vi "SLSC Create Tree Control from EDS datatype.vi"(7 "Property Tree":refnum<vi>, 8 "error in (no error)":errorcluster, 9 "Channel Values":dbl[](array[numeric]), 10 "Properties to enable":string[](array[string]), 11 "SLSC EDS module":T3) -> (0 "error out":errorcluster, 1 "Enum Strings":cluster{"name":string, string}[](array[cluster]), 2 "Enums":T1[](array[typedef]), 3 "SLSC Output Tree":T2(array[cluster])=[{"Left Cell String"="SLSC-12001-030EE1BC-Mod8", "Child Text"=[], "Child Tag"="Device", "Item Indent"=0, "Child Only?"=FALSE, "Glyph Index"=28}, {"Left Cell String"="Commands", "Child Text"=[], "Child Tag"="Device/Commands", "Item Indent"=1, "Child Only?"=FALSE, "Glyph Index"=35}, {"Left Cell String"="NI.UpdateChannelConfiguration", "Child Text"=["", "", "", "", "", "", "Command..NI.UpdateChannelConfiguration", "Command to complete updating physical channel properties", "This command enables simultaneous updating of the functional state of the module's physical channel configuration. Simultaneous updating of the physical channels' properties prevents the register write commit order from creating unexpected channel configuration states. Run this command to make changes to physical channels' properties take effect."], "Child Tag"="Device/Commands/NI.UpdateChannelConfiguration", "Item Indent"=2, "Child Only?"=FALSE, "Glyph Index"=4}, {"Left Cell String"="NI.UpdateTestMode", "Child Text"=["", "", "", "", "", "", "Command..NI.UpdateTestMode", "Command to complete updating Test Mode properties", "This command enable simultaneous updating of the functional state of the module's Test Mode configuration. Run this command to make changes to Test Mode properties take effect."], "Child Tag"="Device/Commands/NI.UpdateTestMode", "Item Indent"=2, "Child Only?"=FALSE, "Glyph Index"=4}, {"Left Cell String"="NI.Acknowledge24VPowerFailed", "Child Text"=["", "", "", "", "", "", "Command..NI.Acknowledge24VPowerFailed", "Command to acknowledge a latched 24V power failure status", "This command tries to clear the module's latched true state for the NI.Status24V_PowerFailed property. This command will have no effect on the latched state if the NI.Status24V_PowerGood property is still false."], "Child Tag"="Device/Commands/NI.Acknowledge24VPowerFailed", "Item Indent"=2, "Child Only?"=FALSE, "Glyph Index"=4}, {"Left Cell String"="Properties", "Child Text"=[], "Child Tag"="Device/Properties", "Item Indent"=1, "Child Only?"=FALSE, "Glyph Index"=36}, {"Left Cell String"="NI.ModuleControllerVersion", "Child Text"=["17022812", "Read Only", "U32", "", "", "", "[3.860173E+8].R.U32..NI.ModuleControllerVersion", "Module Controller Version", "The version is the timestamp, in hexadecimal format, of the time the Module Controller was compiled."], "Child Tag"="Device/Properties/NI.ModuleControllerVersion", "Item Indent"=2, "Child Only?"=FALSE, "Glyph Index"=8}, {"Left Cell String"="NI.RearBufferState", "Child Text"=["0", "Read Only", "U32", "", "", "", "[0].R.U32..NI.RearBufferState", "Logic state of all rear I/O connector input buffers", "Reading this property retrieves the current logic state of the rear I/O connector input buffers. This retrieval is controlled through the software system so the actual sampling time of the inputs is not deterministic. The value at each bit position is a function of the logic state at the XJ2 pin and the corresponding line's direction and enable configuration. An enabled line configured as an input will drive the rear I/O connector input buffer to the same state as detected at the front I/O connector input buffer."], "Child Tag"="Device/Properties/NI.RearBufferState", "Item Indent"=2, "Child Only?"=FALSE, "Glyph Index"=8}, {"Left Cell String"="NI.FrontBufferState", "Child Text"=["0", "Read Only", "U32", "", "", "", "[0].R.U32..NI.FrontBufferState", "Logic state of all front I/O connector input buffers", "Reading this property retrieves the current logic state of the front I/O connector input buffers. This retrieval is controlled through the software system so the actual sampling time of the inputs is not deterministic. The value at each bit position is a function of the voltage at the module DSUB pin and the bank range and threshold configuration. An enabled line configured as an output may drive the front I/O connector input buffer to a specific voltage, depending on the bank supply voltage configuration, the line's output topology, and the line's logic state from the rear I/O connector input buffer."], "Child Tag"="Device/Properties/NI.FrontBufferState", "Item Indent"=2, "Child Only?"=FALSE, "Glyph Index"=8}, {"Left Cell String"="NI.Status24VPowerFailed", "Child Text"=["False", "Read Only", "Bool", "", "", "", "[0].R.Bool..NI.Status24VPowerFailed", "State of the latched failure status of the module's 24V rail from the SLSC Interface", "When the NI.Status24V_PowerGood becomes false, this property latches as true until it is reset by the NI.Status24V_FaultAcknowledge command is sent after NI.Status24V_PowerGood returns to true. If this property is true, then the supply voltage selection for both banks of the module has been forced off for a nonzero duration."], "Child Tag"="Device/Properties/NI.Status24VPowerFailed", "Item Indent"=2, "Child Only?"=FALSE, "Glyph Index"=8}, {"Left Cell String"="NI.Status24VPowerGood", "Child Text"=["True", "Read Only", "Bool", "", "", "", "[1].R.Bool..NI.Status24VPowerGood", "State of the 24V rail on the module from the SLSC Interface", "When the 24V rail from the SLSC Interface drops below the safe operating range for the module, this property is set to false. Simultaneously, to protect the module's output circuitry and to prevent the module front I/O connector outputs from glitching high, the supply voltage selection for both banks is forced off until the 24V rail recovers and is stable."], "Child Tag"="Device/Properties/NI.Status24VPowerGood", "Item Indent"=2, "Child Only?"=FALSE, "Glyph Index"=8}, {"Left Cell String"="NI.Status3_3VPowerGood", "Child Text"=["True", "Read Only", "Bool", "", "", "", "[1].R.Bool..NI.Status3_3VPowerGood", "State of the 3.3V rail from the SLSC Interface on the module", "This property will always be true on a correctly functioning module because the module CPLD requires the 3.3V rail from the SLSC Interface to operate."], "Child Tag"="Device/Properties/NI.Status3_3VPowerGood", "Item Indent"=2, "Child Only?"=FALSE, "Glyph Index"=8}, {"Left Cell String"="NI.TestModeEnable", "Child Text"=["False", "Read/Write", "Bool", "", "", "", "[0].RW.Bool..NI.TestModeEnable", "Enable for Test Mode", "Enable state for the module's Test Mode. When Test Mode is enabled, the module will output the values from the NI.TestModeValue property on the corresponding lines. Each line's respective direction and enable configuration will still apply when Test Mode is active. The data source of the lines is the only change when Test Mode is active. Changes to this property take effect after running the NI.TestModeUpdate command."], "Child Tag"="Device/Properties/NI.TestModeEnable", "Item Indent"=2, "Child Only?"=FALSE, "Glyph Index"=9}, {"Left Cell String"="NI.TestModeValue", "Child Text"=["0", "Read/Write", "U32", "", "", "", "[0].RW.U32..NI.TestModeValue", "Output logic states for use during Test Mode", "Output logic states for the module for use during Test Mode. The logic state corresponding to each line may be set independently of the other states. Changes to this property take effect after running the NI.TestModeUpdate command."], "Child Tag"="Device/Properties/NI.TestModeValue", "Item Indent"=2, "Child Only?"=FALSE, "Glyph Index"=9}, {"Left Cell String"="SLSC-12001-030EE1BC-Mod8/bank0", "Child Text"=[], "Child Tag"="Physical Channel/bank0", "Item Indent"=1, "Child Only?"=FALSE, "Glyph Index"=31}, {"Left Cell String"="Commands", "Child Text"=[], "Child Tag"="Physical Channel/bank0/Commands", "Item Indent"=2, "Child Only?"=FALSE, "Glyph Index"=35}, {"Left Cell String"="Properties", "Child Text"=[], "Child Tag"="Physical Channel/bank0/Properties", "Item Indent"=2, "Child Only?"=FALSE, "Glyph Index"=36}, {"Left Cell String"="NI.VsupSelect", "Child Text"=["[0]Vsup_Off", "Read/Write", "I32", "Enum", "NI.VsupSource", "[0]Vsup_Off;[1]Vsup_0;[2]Vsup_1;", "[0].RW.I32.bank0.NI.VsupSelect", "Voltage source selection", "Voltage source selection for this bank. Changes to this property take effect after running the NI.ChannelConfigurationUpdate command."], "Child Tag"="Physical Channel/bank0/Properties/NI.VsupSelect", "Item Indent"=3, "Child Only?"=FALSE, "Glyph Index"=9}, {"Left Cell String"="NI.RangeEnable5V", "Child Text"=["False", "Read/Write", "Bool", "", "", "", "[0].RW.Bool.bank0.NI.RangeEnable5V", "Voltage range selection", "Enable state for this bank's voltage range. When enabled, this bank uses the NI.InputThreshold5V for the input threshold. When disabled, this bank uses the NI.InputThreshold33V for the input threshold. Changes to this property take effect after running the NI.ChannelConfigurationUpdate command."], "Child Tag"="Physical Channel/bank0/Properties/NI.RangeEnable5V", "Item Indent"=3, "Child Only?"=FALSE, "Glyph Index"=9}, {"Left Cell String"="NI.InputThreshold5V", "Child Text"=["0.7", "Read/Write", "DBL", "", "", "", "[0.7].RW.DBL.bank0.NI.InputThreshold5V", "Input threshold voltage for the 5 V range", "Input threshold voltage for this bank when its NI.RangeEnable5V is true. Changes to this property take effect after running the NI.ChannelConfigurationUpdate command."], "Child Tag"="Physical Channel/bank0/Properties/NI.InputThreshold5V", "Item Indent"=3, "Child Only?"=FALSE, "Glyph Index"=9}, {"Left Cell String"="NI.InputThreshold33V", "Child Text"=["3.706", "Read/Write", "DBL", "", "", "", "[3.706].RW.DBL.bank0.NI.InputThreshold33V", "Input threshold voltage for the 33 V range", "Input threshold voltage for this bank when its NI.RangeEnable5V is false. Changes to this property take effect after running the NI.ChannelConfigurationUpdate command."], "Child Tag"="Physical Channel/bank0/Properties/NI.InputThreshold33V", "Item Indent"=3, "Child Only?"=FALSE, "Glyph Index"=9}, {"Left Cell String"="SLSC-12001-030EE1BC-Mod8/bank1", "Child Text"=[], "Child Tag"="Physical Channel/bank1", "Item Indent"=1, "Child Only?"=FALSE, "Glyph Index"=31}, {"Left Cell String"="Commands", "Child Text"=[], "Child Tag"="Physical Channel/bank1/Commands", "Item Indent"=2, "Child Only?"=FALSE, "Glyph Index"=35}, {"Left Cell String"="Properties", "Child Text"=[], "Child Tag"="Physical Channel/bank1/Properties", "Item Indent"=2, "Child Only?"=FALSE, "Glyph Index"=36}, {"Left Cell String"="NI.VsupSelect", "Child Text"=["[0]Vsup_Off", "Read/Write", "I32", "Enum", "NI.VsupSource", "[0]Vsup_Off;[1]Vsup_0;[2]Vsup_1;", "[0].RW.I32.bank1.NI.VsupSelect", "Voltage source selection", "Voltage source selection for this bank. Changes to this property take effect after running the NI.ChannelConfigurationUpdate command."], "Child Tag"="Physical Channel/bank1/Properties/NI.VsupSelect", "Item Indent"=3, "Child Only?"=FALSE, "Glyph Index"=9}, {"Left Cell String"="NI.RangeEnable5V", "Child Text"=["False", "Read/Write", "Bool", "", "", "", "[0].RW.Bool.bank1.NI.RangeEnable5V", "Voltage range selection", "Enable state for this bank's voltage range. When enabled, this bank uses the NI.InputThreshold5V for the input threshold. When disabled, this bank uses the NI.InputThreshold33V for the input threshold. Changes to this property take effect after running the NI.ChannelConfigurationUpdate command."], "Child Tag"="Physical Channel/bank1/Properties/NI.RangeEnable5V", "Item Indent"=3, "Child Only?"=FALSE, "Glyph Index"=9}, {"Left Cell String"="NI.InputThreshold5V", "Child Text"=["0.7", "Read/Write", "DBL", "", "", "", "[0.7].RW.DBL.bank1.NI.InputThreshold5V", "Input threshold voltage for the 5 V range", "Input threshold voltage for this bank when its NI.RangeEnable5V is true. Changes to this property take effect after running the NI.ChannelConfigurationUpdate command."], "Child Tag"="Physical Channel/bank1/Properties/NI.InputThreshold5V", "Item Indent"=3, "Child Only?"=FALSE, "Glyph Index"=9}, {"Left Cell String"="NI.InputThreshold33V", "Child Text"=["3.706", "Read/Write", "DBL", "", "", "", "[3.706].RW.DBL.bank1.NI.InputThreshold33V", "Input threshold voltage for the 33 V range", "Input threshold voltage for this bank when its NI.RangeEnable5V is false. Changes to this property take effect after running the NI.ChannelConfigurationUpdate command."], "Child Tag"="Physical Channel/bank1/Properties/NI.InputThreshold33V", "Item Indent"=3, "Child Only?"=FALSE, "Glyph Index"=9}, {"Left Cell String"="SLSC-12001-030EE1BC-Mod8/port0/line0", "Child Text"=[], "Child Tag"="Physical Channel/port0/line0", "Item Indent"=1, "Child Only?"=FALSE, "Glyph Index"=31}, {"Left Cell String"="Commands", "Child Text"=[], "Child Tag"="Physical Channel/port0/line0/Commands", "Item Indent"=2, "Child Only?"=FALSE, "Glyph Index"=35}, {"Left Cell String"="Properties", "Child Text"=[], "Child Tag"="Physical Channel/port0/line0/Properties", "Item Indent"=2, "Child Only?"=FALSE, "Glyph Index"=36}, {"Left Cell String"="NI.Line.Index", "Child Text"=["0", "Read Only", "U32", "", "", "", "[0].R.U32.port0/line0.NI.Line.Index", "Overall index of this DIO line in the module", "This is the index of this DIO line for the aggregate module properties: NI.FrontInputBufferState, NI.RearInputBufferState, and NI.TestModeValue."], "Child Tag"="Physical Channel/port0/line0/Properties/NI.Line.Index", "Item Indent"=3, "Child Only?"=FALSE, "Glyph Index"=8}, {"Left Cell String"="NI.Line.Direction", "Child Text"=["[0]Input", "Read/Write", "I32", "Enum", "NI.Line.Direction", "[0]Input;[1]Output_Source;[2]Output_Sink;[3]Output_PushPull;", "[0].RW.I32.port0/line0.NI.Line.Direction", "DIO line direction", "Line signal flow direction through the module, relative to the front I/O connector. This property is only used when the NI.ChannelEnable for this line is set to true. Changes to this property take effect after running the NI.ChannelConfigurationUpdate command."], "Child Tag"="Physical Channel/port0/line0/Properties/NI.Line.Direction", "Item Indent"=3, "Child Only?"=FALSE, "Glyph Index"=9}, {"Left Cell String"="NI.Line.Enable", "Child Text"=["False", "Read/Write", "Bool", "", "", "", "[0].RW.Bool.port0/line0.NI.Line.Enable", "DIO line output enable", "DIO output enable for one line. When a line is enabled, the input and output buffers for the front I/O connector and the rear I/O connector of the line are configured based on the NI.Line.Direction property. When a line is not enabled, the buffers for both the front I/O connector and the rear I/O connector are configured as inputs. Changes to this property take effect after running the NI.ChannelConfigurationUpdate command."], "Child Tag"="Physical Channel/port0/line0/Properties/NI.Line.Enable", "Item Indent"=3, "Child Only?"=FALSE, "Glyph Index"=9}, {"Left Cell String"="SLSC-12001-030EE1BC-Mod8/port0/line1", "Child Text"=[], "Child Tag"="Physical Channel/port0/line1", "Item Indent"=1, "Child Only?"=FALSE, "Glyph Index"=31}, {"Left Cell String"="Commands", "Child Text"=[], "Child Tag"="Physical Channel/port0/line1/Commands", "Item Indent"=2, "Child Only?"=FALSE, "Glyph Index"=35}, {"Left Cell String"="Properties", "Child Text"=[], "Child Tag"="Physical Channel/port0/line1/Properties", "Item Indent"=2, "Child Only?"=FALSE, "Glyph Index"=36}, {"Left Cell String"="NI.Line.Index", "Child Text"=["1", "Read Only", "U32", "", "", "", "[1].R.U32.port0/line1.NI.Line.Index", "Overall index of this DIO line in the module", "This is the index of this DIO line for the aggregate module properties: NI.FrontInputBufferState, NI.RearInputBufferState, and NI.TestModeValue."], "Child Tag"="Physical Channel/port0/line1/Properties/NI.Line.Index", "Item Indent"=3, "Child Only?"=FALSE, "Glyph Index"=8}, {"Left Cell String"="NI.Line.Direction", "Child Text"=["[0]Input", "Read/Write", "I32", "Enum", "NI.Line.Direction", "[0]Input;[1]Output_Source;[2]Output_Sink;[3]Output_PushPull;", "[0].RW.I32.port0/line1.NI.Line.Direction", "DIO line direction", "Line signal flow direction through the module, relative to the front I/O connector. This property is only used when the NI.ChannelEnable for this line is set to true. Changes to this property take effect after running the NI.ChannelConfigurationUpdate command."], "Child Tag"="Physical Channel/port0/line1/Properties/NI.Line.Direction", "Item Indent"=3, "Child Only?"=FALSE, "Glyph Index"=9}, {"Left Cell String"="NI.Line.Enable", "Child Text"=["False", "Read/Write", "Bool", "", "", "", "[0].RW.Bool.port0/line1.NI.Line.Enable", "DIO line output enable", "DIO output enable for one line. When a line is enabled, the input and output buffers for the front I/O connector and the rear I/O connector of the line are configured based on the NI.Line.Direction property. When a line is not enabled, the buffers for both the front I/O connector and the rear I/O connector are configured as inputs. Changes to this property take effect after running the NI.ChannelConfigurationUpdate command."], "Child Tag"="Physical Channel/port0/line1/Properties/NI.Line.Enable", "Item Indent"=3, "Child Only?"=FALSE, "Glyph Index"=9}, {"Left Cell String"="SLSC-12001-030EE1BC-Mod8/port0/line2", "Child Text"=[], "Child Tag"="Physical Channel/port0/line2", "Item Indent"=1, "Child Only?"=FALSE, "Glyph Index"=31}, {"Left Cell String"="Commands", "Child Text"=[], "Child Tag"="Physical Channel/port0/line2/Commands", "Item Indent"=2, "Child Only?"=FALSE, "Glyph Index"=35}, {"Left Cell String"="Properties", "Child Text"=[], "Child Tag"="Physical Channel/port0/line2/Properties", "Item Indent"=2, "Child Only?"=FALSE, "Glyph Index"=36}, {"Left Cell String"="NI.Line.Index", "Child Text"=["2", "Read Only", "U32", "", "", "", "[2].R.U32.port0/line2.NI.Line.Index", "Overall index of this DIO line in the module", "This is the index of this DIO line for the aggregate module properties: NI.FrontInputBufferState, NI.RearInputBufferState, and NI.TestModeValue."], "Child Tag"="Physical Channel/port0/line2/Properties/NI.Line.Index", "Item Indent"=3, "Child Only?"=FALSE, "Glyph Index"=8}, {"Left Cell String"="NI.Line.Direction", "Child Text"=["[0]Input", "Read/Write", "I32", "Enum", "NI.Line.Direction", "[0]Input;[1]Output_Source;[2]Output_Sink;[3]Output_PushPull;", "[0].RW.I32.port0/line2.NI.Line.Direction", "DIO line direction", "Line signal flow direction through the module, relative to the front I/O connector. This property is only used when the NI.ChannelEnable for this line is set to true. Changes to this property take effect after running the NI.ChannelConfigurationUpdate command."], "Child Tag"="Physical Channel/port0/line2/Properties/NI.Line.Direction", "Item Indent"=3, "Child Only?"=FALSE, "Glyph Index"=9}, {"Left Cell String"="NI.Line.Enable", "Child Text"=["False", "Read/Write", "Bool", "", "", "", "[0].RW.Bool.port0/line2.NI.Line.Enable", "DIO line output enable", "DIO output enable for one line. When a line is enabled, the input and output buffers for the front I/O connector and the rear I/O connector of the line are configured based on the NI.Line.Direction property. When a line is not enabled, the buffers for both the front I/O connector and the rear I/O connector are configured as inputs. Changes to this property take effect after running the NI.ChannelConfigurationUpdate command."], "Child Tag"="Physical Channel/port0/line2/Properties/NI.Line.Enable", "Item Indent"=3, "Child Only?"=FALSE, "Glyph Index"=9}, {"Left Cell String"="SLSC-12001-030EE1BC-Mod8/port0/line3", "Child Text"=[], "Child Tag"="Physical Channel/port0/line3", "Item Indent"=1, "Child Only?"=FALSE, "Glyph Index"=31}, {"Left Cell String"="Commands", "Child Text"=[], "Child Tag"="Physical Channel/port0/line3/Commands", "Item Indent"=2, "Child Only?"=FALSE, "Glyph Index"=35}, {"Left Cell String"="Properties", "Child Text"=[], "Child Tag"="Physical Channel/port0/line3/Properties", "Item Indent"=2, "Child Only?"=FALSE, "Glyph Index"=36}, {"Left Cell String"="NI.Line.Index", "Child Text"=["3", "Read Only", "U32", "", "", "", "[3].R.U32.port0/line3.NI.Line.Index", "Overall index of this DIO line in the module", "This is the index of this DIO line for the aggregate module properties: NI.FrontInputBufferState, NI.RearInputBufferState, and NI.TestModeValue."], "Child Tag"="Physical Channel/port0/line3/Properties/NI.Line.Index", "Item Indent"=3, "Child Only?"=FALSE, "Glyph Index"=8}, {"Left Cell String"="NI.Line.Direction", "Child Text"=["[0]Input", "Read/Write", "I32", "Enum", "NI.Line.Direction", "[0]Input;[1]Output_Source;[2]Output_Sink;[3]Output_PushPull;", "[0].RW.I32.port0/line3.NI.Line.Direction", "DIO line direction", "Line signal flow direction through the module, relative to the front I/O connector. This property is only used when the NI.ChannelEnable for this line is set to true. Changes to this property take effect after running the NI.ChannelConfigurationUpdate command."], "Child Tag"="Physical Channel/port0/line3/Properties/NI.Line.Direction", "Item Indent"=3, "Child Only?"=FALSE, "Glyph Index"=9}, {"Left Cell String"="NI.Line.Enable", "Child Text"=["False", "Read/Write", "Bool", "", "", "", "[0].RW.Bool.port0/line3.NI.Line.Enable", "DIO line output enable", "DIO output enable for one line. When a line is enabled, the input and output buffers for the front I/O connector and the rear I/O connector of the line are configured based on the NI.Line.Direction property. When a line is not enabled, the buffers for both the front I/O connector and the rear I/O connector are configured as inputs. Changes to this property take effect after running the NI.ChannelConfigurationUpdate command."], "Child Tag"="Physical Channel/port0/line3/Properties/NI.Line.Enable", "Item Indent"=3, "Child Only?"=FALSE, "Glyph Index"=9}, {"Left Cell String"="SLSC-12001-030EE1BC-Mod8/port0/line4", "Child Text"=[], "Child Tag"="Physical Channel/port0/line4", "Item Indent"=1, "Child Only?"=FALSE, "Glyph Index"=31}, {"Left Cell String"="Commands", "Child Text"=[], "Child Tag"="Physical Channel/port0/line4/Commands", "Item Indent"=2, "Child Only?"=FALSE, "Glyph Index"=35}, {"Left Cell String"="Properties", "Child Text"=[], "Child Tag"="Physical Channel/port0/line4/Properties", "Item Indent"=2, "Child Only?"=FALSE, "Glyph Index"=36}, {"Left Cell String"="NI.Line.Index", "Child Text"=["4", "Read Only", "U32", "", "", "", "[4].R.U32.port0/line4.NI.Line.Index", "Overall index of this DIO line in the module", "This is the index of this DIO line for the aggregate module properties: NI.FrontInputBufferState, NI.RearInputBufferState, and NI.TestModeValue."], "Child Tag"="Physical Channel/port0/line4/Properties/NI.Line.Index", "Item Indent"=3, "Child Only?"=FALSE, "Glyph Index"=8}, {"Left Cell String"="NI.Line.Direction", "Child Text"=["[0]Input", "Read/Write", "I32", "Enum", "NI.Line.Direction", "[0]Input;[1]Output_Source;[2]Output_Sink;[3]Output_PushPull;", "[0].RW.I32.port0/line4.NI.Line.Direction", "DIO line direction", "Line signal flow direction through the module, relative to the front I/O connector. This property is only used when the NI.ChannelEnable for this line is set to true. Changes to this property take effect after running the NI.ChannelConfigurationUpdate command."], "Child Tag"="Physical Channel/port0/line4/Properties/NI.Line.Direction", "Item Indent"=3, "Child Only?"=FALSE, "Glyph Index"=9}, {"Left Cell String"="NI.Line.Enable", "Child Text"=["False", "Read/Write", "Bool", "", "", "", "[0].RW.Bool.port0/line4.NI.Line.Enable", "DIO line output enable", "DIO output enable for one line. When a line is enabled, the input and output buffers for the front I/O connector and the rear I/O connector of the line are configured based on the NI.Line.Direction property. When a line is not enabled, the buffers for both the front I/O connector and the rear I/O connector are configured as inputs. Changes to this property take effect after running the NI.ChannelConfigurationUpdate command."], "Child Tag"="Physical Channel/port0/line4/Properties/NI.Line.Enable", "Item Indent"=3, "Child Only?"=FALSE, "Glyph Index"=9}, {"Left Cell String"="SLSC-12001-030EE1BC-Mod8/port0/line5", "Child Text"=[], "Child Tag"="Physical Channel/port0/line5", "Item Indent"=1, "Child Only?"=FALSE, "Glyph Index"=31}, {"Left Cell String"="Commands", "Child Text"=[], "Child Tag"="Physical Channel/port0/line5/Commands", "Item Indent"=2, "Child Only?"=FALSE, "Glyph Index"=35}, {"Left Cell String"="Properties", "Child Text"=[], "Child Tag"="Physical Channel/port0/line5/Properties", "Item Indent"=2, "Child Only?"=FALSE, "Glyph Index"=36}, {"Left Cell String"="NI.Line.Index", "Child Text"=["5", "Read Only", "U32", "", "", "", "[5].R.U32.port0/line5.NI.Line.Index", "Overall index of this DIO line in the module", "This is the index of this DIO line for the aggregate module properties: NI.FrontInputBufferState, NI.RearInputBufferState, and NI.TestModeValue."], "Child Tag"="Physical Channel/port0/line5/Properties/NI.Line.Index", "Item Indent"=3, "Child Only?"=FALSE, "Glyph Index"=8}, {"Left Cell String"="NI.Line.Direction", "Child Text"=["[0]Input", "Read/Write", "I32", "Enum", "NI.Line.Direction", "[0]Input;[1]Output_Source;[2]Output_Sink;[3]Output_PushPull;", "[0].RW.I32.port0/line5.NI.Line.Direction", "DIO line direction", "Line signal flow direction through the module, relative to the front I/O connector. This property is only used when the NI.ChannelEnable for this line is set to true. Changes to this property take effect after running the NI.ChannelConfigurationUpdate command."], "Child Tag"="Physical Channel/port0/line5/Properties/NI.Line.Direction", "Item Indent"=3, "Child Only?"=FALSE, "Glyph Index"=9}, {"Left Cell String"="NI.Line.Enable", "Child Text"=["False", "Read/Write", "Bool", "", "", "", "[0].RW.Bool.port0/line5.NI.Line.Enable", "DIO line output enable", "DIO output enable for one line. When a line is enabled, the input and output buffers for the front I/O connector and the rear I/O connector of the line are configured based on the NI.Line.Direction property. When a line is not enabled, the buffers for both the front I/O connector and the rear I/O connector are configured as inputs. Changes to this property take effect after running the NI.ChannelConfigurationUpdate command."], "Child Tag"="Physical Channel/port0/line5/Properties/NI.Line.Enable", "Item Indent"=3, "Child Only?"=FALSE, "Glyph Index"=9}, {"Left Cell String"="SLSC-12001-030EE1BC-Mod8/port0/line6", "Child Text"=[], "Child Tag"="Physical Channel/port0/line6", "Item Indent"=1, "Child Only?"=FALSE, "Glyph Index"=31}, {"Left Cell String"="Commands", "Child Text"=[], "Child Tag"="Physical Channel/port0/line6/Commands", "Item Indent"=2, "Child Only?"=FALSE, "Glyph Index"=35}, {"Left Cell String"="Properties", "Child Text"=[], "Child Tag"="Physical Channel/port0/line6/Properties", "Item Indent"=2, "Child Only?"=FALSE, "Glyph Index"=36}, {"Left Cell String"="NI.Line.Index", "Child Text"=["6", "Read Only", "U32", "", "", "", "[6].R.U32.port0/line6.NI.Line.Index", "Overall index of this DIO line in the module", "This is the index of this DIO line for the aggregate module properties: NI.FrontInputBufferState, NI.RearInputBufferState, and NI.TestModeValue."], "Child Tag"="Physical Channel/port0/line6/Properties/NI.Line.Index", "Item Indent"=3, "Child Only?"=FALSE, "Glyph Index"=8}, {"Left Cell String"="NI.Line.Direction", "Child Text"=["[0]Input", "Read/Write", "I32", "Enum", "NI.Line.Direction", "[0]Input;[1]Output_Source;[2]Output_Sink;[3]Output_PushPull;", "[0].RW.I32.port0/line6.NI.Line.Direction", "DIO line direction", "Line signal flow direction through the module, relative to the front I/O connector. This property is only used when the NI.ChannelEnable for this line is set to true. Changes to this property take effect after running the NI.ChannelConfigurationUpdate command."], "Child Tag"="Physical Channel/port0/line6/Properties/NI.Line.Direction", "Item Indent"=3, "Child Only?"=FALSE, "Glyph Index"=9}, {"Left Cell String"="NI.Line.Enable", "Child Text"=["False", "Read/Write", "Bool", "", "", "", "[0].RW.Bool.port0/line6.NI.Line.Enable", "DIO line output enable", "DIO output enable for one line. When a line is enabled, the input and output buffers for the front I/O connector and the rear I/O connector of the line are configured based on the NI.Line.Direction property. When a line is not enabled, the buffers for both the front I/O connector and the rear I/O connector are configured as inputs. Changes to this property take effect after running the NI.ChannelConfigurationUpdate command."], "Child Tag"="Physical Channel/port0/line6/Properties/NI.Line.Enable", "Item Indent"=3, "Child Only?"=FALSE, "Glyph Index"=9}, {"Left Cell String"="SLSC-12001-030EE1BC-Mod8/port0/line7", "Child Text"=[], "Child Tag"="Physical Channel/port0/line7", "Item Indent"=1, "Child Only?"=FALSE, "Glyph Index"=31}, {"Left Cell String"="Commands", "Child Text"=[], "Child Tag"="Physical Channel/port0/line7/Commands", "Item Indent"=2, "Child Only?"=FALSE, "Glyph Index"=35}, {"Left Cell String"="Properties", "Child Text"=[], "Child Tag"="Physical Channel/port0/line7/Properties", "Item Indent"=2, "Child Only?"=FALSE, "Glyph Index"=36}, {"Left Cell String"="NI.Line.Index", "Child Text"=["7", "Read Only", "U32", "", "", "", "[7].R.U32.port0/line7.NI.Line.Index", "Overall index of this DIO line in the module", "This is the index of this DIO line for the aggregate module properties: NI.FrontInputBufferState, NI.RearInputBufferState, and NI.TestModeValue."], "Child Tag"="Physical Channel/port0/line7/Properties/NI.Line.Index", "Item Indent"=3, "Child Only?"=FALSE, "Glyph Index"=8}, {"Left Cell String"="NI.Line.Direction", "Child Text"=["[0]Input", "Read/Write", "I32", "Enum", "NI.Line.Direction", "[0]Input;[1]Output_Source;[2]Output_Sink;[3]Output_PushPull;", "[0].RW.I32.port0/line7.NI.Line.Direction", "DIO line direction", "Line signal flow direction through the module, relative to the front I/O connector. This property is only used when the NI.ChannelEnable for this line is set to true. Changes to this property take effect after running the NI.ChannelConfigurationUpdate command."], "Child Tag"="Physical Channel/port0/line7/Properties/NI.Line.Direction", "Item Indent"=3, "Child Only?"=FALSE, "Glyph Index"=9}, {"Left Cell String"="NI.Line.Enable", "Child Text"=["False", "Read/Write", "Bool", "", "", "", "[0].RW.Bool.port0/line7.NI.Line.Enable", "DIO line output enable", "DIO output enable for one line. When a line is enabled, the input and output buffers for the front I/O connector and the rear I/O connector of the line are configured based on the NI.Line.Direction property. When a line is not enabled, the buffers for both the front I/O connector and the rear I/O connector are configured as inputs. Changes to this property take effect after running the NI.ChannelConfigurationUpdate command."], "Child Tag"="Physical Channel/port0/line7/Properties/NI.Line.Enable", "Item Indent"=3, "Child Only?"=FALSE, "Glyph Index"=9}, {"Left Cell String"="SLSC-12001-030EE1BC-Mod8/port1/line0", "Child Text"=[], "Child Tag"="Physical Channel/port1/line0", "Item Indent"=1, "Child Only?"=FALSE, "Glyph Index"=31}, {"Left Cell String"="Commands", "Child Text"=[], "Child Tag"="Physical Channel/port1/line0/Commands", "Item Indent"=2, "Child Only?"=FALSE, "Glyph Index"=35}, {"Left Cell String"="Properties", "Child Text"=[], "Child Tag"="Physical Channel/port1/line0/Properties", "Item Indent"=2, "Child Only?"=FALSE, "Glyph Index"=36}, {"Left Cell String"="NI.Line.Index", "Child Text"=["8", "Read Only", "U32", "", "", "", "[8].R.U32.port1/line0.NI.Line.Index", "Overall index of this DIO line in the module", "This is the index of this DIO line for the aggregate module properties: NI.FrontInputBufferState, NI.RearInputBufferState, and NI.TestModeValue."], "Child Tag"="Physical Channel/port1/line0/Properties/NI.Line.Index", "Item Indent"=3, "Child Only?"=FALSE, "Glyph Index"=8}, {"Left Cell String"="NI.Line.Direction", "Child Text"=["[0]Input", "Read/Write", "I32", "Enum", "NI.Line.Direction", "[0]Input;[1]Output_Source;[2]Output_Sink;[3]Output_PushPull;", "[0].RW.I32.port1/line0.NI.Line.Direction", "DIO line direction", "Line signal flow direction through the module, relative to the front I/O connector. This property is only used when the NI.ChannelEnable for this line is set to true. Changes to this property take effect after running the NI.ChannelConfigurationUpdate command."], "Child Tag"="Physical Channel/port1/line0/Properties/NI.Line.Direction", "Item Indent"=3, "Child Only?"=FALSE, "Glyph Index"=9}, {"Left Cell String"="NI.Line.Enable", "Child Text"=["False", "Read/Write", "Bool", "", "", "", "[0].RW.Bool.port1/line0.NI.Line.Enable", "DIO line output enable", "DIO output enable for one line. When a line is enabled, the input and output buffers for the front I/O connector and the rear I/O connector of the line are configured based on the NI.Line.Direction property. When a line is not enabled, the buffers for both the front I/O connector and the rear I/O connector are configured as inputs. Changes to this property take effect after running the NI.ChannelConfigurationUpdate command."], "Child Tag"="Physical Channel/port1/line0/Properties/NI.Line.Enable", "Item Indent"=3, "Child Only?"=FALSE, "Glyph Index"=9}, {"Left Cell String"="SLSC-12001-030EE1BC-Mod8/port1/line1", "Child Text"=[], "Child Tag"="Physical Channel/port1/line1", "Item Indent"=1, "Child Only?"=FALSE, "Glyph Index"=31}, {"Left Cell String"="Commands", "Child Text"=[], "Child Tag"="Physical Channel/port1/line1/Commands", "Item Indent"=2, "Child Only?"=FALSE, "Glyph Index"=35}, {"Left Cell String"="Properties", "Child Text"=[], "Child Tag"="Physical Channel/port1/line1/Properties", "Item Indent"=2, "Child Only?"=FALSE, "Glyph Index"=36}, {"Left Cell String"="NI.Line.Index", "Child Text"=["9", "Read Only", "U32", "", "", "", "[9].R.U32.port1/line1.NI.Line.Index", "Overall index of this DIO line in the module", "This is the index of this DIO line for the aggregate module properties: NI.FrontInputBufferState, NI.RearInputBufferState, and NI.TestModeValue."], "Child Tag"="Physical Channel/port1/line1/Properties/NI.Line.Index", "Item Indent"=3, "Child Only?"=FALSE, "Glyph Index"=8}, {"Left Cell String"="NI.Line.Direction", "Child Text"=["[0]Input", "Read/Write", "I32", "Enum", "NI.Line.Direction", "[0]Input;[1]Output_Source;[2]Output_Sink;[3]Output_PushPull;", "[0].RW.I32.port1/line1.NI.Line.Direction", "DIO line direction", "Line signal flow direction through the module, relative to the front I/O connector. This property is only used when the NI.ChannelEnable for this line is set to true. Changes to this property take effect after running the NI.ChannelConfigurationUpdate command."], "Child Tag"="Physical Channel/port1/line1/Properties/NI.Line.Direction", "Item Indent"=3, "Child Only?"=FALSE, "Glyph Index"=9}, {"Left Cell String"="NI.Line.Enable", "Child Text"=["False", "Read/Write", "Bool", "", "", "", "[0].RW.Bool.port1/line1.NI.Line.Enable", "DIO line output enable", "DIO output enable for one line. When a line is enabled, the input and output buffers for the front I/O connector and the rear I/O connector of the line are configured based on the NI.Line.Direction property. When a line is not enabled, the buffers for both the front I/O connector and the rear I/O connector are configured as inputs. Changes to this property take effect after running the NI.ChannelConfigurationUpdate command."], "Child Tag"="Physical Channel/port1/line1/Properties/NI.Line.Enable", "Item Indent"=3, "Child Only?"=FALSE, "Glyph Index"=9}, {"Left Cell String"="SLSC-12001-030EE1BC-Mod8/port1/line2", "Child Text"=[], "Child Tag"="Physical Channel/port1/line2", "Item Indent"=1, "Child Only?"=FALSE, "Glyph Index"=31}, {"Left Cell String"="Commands", "Child Text"=[], "Child Tag"="Physical Channel/port1/line2/Commands", "Item Indent"=2, "Child Only?"=FALSE, "Glyph Index"=35}, {"Left Cell String"="Properties", "Child Text"=[], "Child Tag"="Physical Channel/port1/line2/Properties", "Item Indent"=2, "Child Only?"=FALSE, "Glyph Index"=36}, {"Left Cell String"="NI.Line.Index", "Child Text"=["A", "Read Only", "U32", "", "", "", "[10].R.U32.port1/line2.NI.Line.Index", "Overall index of this DIO line in the module", "This is the index of this DIO line for the aggregate module properties: NI.FrontInputBufferState, NI.RearInputBufferState, and NI.TestModeValue."], "Child Tag"="Physical Channel/port1/line2/Properties/NI.Line.Index", "Item Indent"=3, "Child Only?"=FALSE, "Glyph Index"=8}, {"Left Cell String"="NI.Line.Direction", "Child Text"=["[0]Input", "Read/Write", "I32", "Enum", "NI.Line.Direction", "[0]Input;[1]Output_Source;[2]Output_Sink;[3]Output_PushPull;", "[0].RW.I32.port1/line2.NI.Line.Direction", "DIO line direction", "Line signal flow direction through the module, relative to the front I/O connector. This property is only used when the NI.ChannelEnable for this line is set to true. Changes to this property take effect after running the NI.ChannelConfigurationUpdate command."], "Child Tag"="Physical Channel/port1/line2/Properties/NI.Line.Direction", "Item Indent"=3, "Child Only?"=FALSE, "Glyph Index"=9}, {"Left Cell String"="NI.Line.Enable", "Child Text"=["False", "Read/Write", "Bool", "", "", "", "[0].RW.Bool.port1/line2.NI.Line.Enable", "DIO line output enable", "DIO output enable for one line. When a line is enabled, the input and output buffers for the front I/O connector and the rear I/O connector of the line are configured based on the NI.Line.Direction property. When a line is not enabled, the buffers for both the front I/O connector and the rear I/O connector are configured as inputs. Changes to this property take effect after running the NI.ChannelConfigurationUpdate command."], "Child Tag"="Physical Channel/port1/line2/Properties/NI.Line.Enable", "Item Indent"=3, "Child Only?"=FALSE, "Glyph Index"=9}, {"Left Cell String"="SLSC-12001-030EE1BC-Mod8/port1/line3", "Child Text"=[], "Child Tag"="Physical Channel/port1/line3", "Item Indent"=1, "Child Only?"=FALSE, "Glyph Index"=31}, {"Left Cell String"="Commands", "Child Text"=[], "Child Tag"="Physical Channel/port1/line3/Commands", "Item Indent"=2, "Child Only?"=FALSE, "Glyph Index"=35}, {"Left Cell String"="Properties", "Child Text"=[], "Child Tag"="Physical Channel/port1/line3/Properties", "Item Indent"=2, "Child Only?"=FALSE, "Glyph Index"=36}, {"Left Cell String"="NI.Line.Index", "Child Text"=["B", "Read Only", "U32", "", "", "", "[11].R.U32.port1/line3.NI.Line.Index", "Overall index of this DIO line in the module", "This is the index of this DIO line for the aggregate module properties: NI.FrontInputBufferState, NI.RearInputBufferState, and NI.TestModeValue."], "Child Tag"="Physical Channel/port1/line3/Properties/NI.Line.Index", "Item Indent"=3, "Child Only?"=FALSE, "Glyph Index"=8}, {"Left Cell String"="NI.Line.Direction", "Child Text"=["[0]Input", "Read/Write", "I32", "Enum", "NI.Line.Direction", "[0]Input;[1]Output_Source;[2]Output_Sink;[3]Output_PushPull;", "[0].RW.I32.port1/line3.NI.Line.Direction", "DIO line direction", "Line signal flow direction through the module, relative to the front I/O connector. This property is only used when the NI.ChannelEnable for this line is set to true. Changes to this property take effect after running the NI.ChannelConfigurationUpdate command."], "Child Tag"="Physical Channel/port1/line3/Properties/NI.Line.Direction", "Item Indent"=3, "Child Only?"=FALSE, "Glyph Index"=9}, {"Left Cell String"="NI.Line.Enable", "Child Text"=["False", "Read/Write", "Bool", "", "", "", "[0].RW.Bool.port1/line3.NI.Line.Enable", "DIO line output enable", "DIO output enable for one line. When a line is enabled, the input and output buffers for the front I/O connector and the rear I/O connector of the line are configured based on the NI.Line.Direction property. When a line is not enabled, the buffers for both the front I/O connector and the rear I/O connector are configured as inputs. Changes to this property take effect after running the NI.ChannelConfigurationUpdate command."], "Child Tag"="Physical Channel/port1/line3/Properties/NI.Line.Enable", "Item Indent"=3, "Child Only?"=FALSE, "Glyph Index"=9}, {"Left Cell String"="SLSC-12001-030EE1BC-Mod8/port1/line4", "Child Text"=[], "Child Tag"="Physical Channel/port1/line4", "Item Indent"=1, "Child Only?"=FALSE, "Glyph Index"=31}, {"Left Cell String"="Commands", "Child Text"=[], "Child Tag"="Physical Channel/port1/line4/Commands", "Item Indent"=2, "Child Only?"=FALSE, "Glyph Index"=35}, {"Left Cell String"="Properties", "Child Text"=[], "Child Tag"="Physical Channel/port1/line4/Properties", "Item Indent"=2, "Child Only?"=FALSE, "Glyph Index"=36}, {"Left Cell String"="NI.Line.Index", "Child Text"=["C", "Read Only", "U32", "", "", "", "[12].R.U32.port1/line4.NI.Line.Index", "Overall index of this DIO line in the module", "This is the index of this DIO line for the aggregate module properties: NI.FrontInputBufferState, NI.RearInputBufferState, and NI.TestModeValue."], "Child Tag"="Physical Channel/port1/line4/Properties/NI.Line.Index", "Item Indent"=3, "Child Only?"=FALSE, "Glyph Index"=8}, {"Left Cell String"="NI.Line.Direction", "Child Text"=["[0]Input", "Read/Write", "I32", "Enum", "NI.Line.Direction", "[0]Input;[1]Output_Source;[2]Output_Sink;[3]Output_PushPull;", "[0].RW.I32.port1/line4.NI.Line.Direction", "DIO line direction", "Line signal flow direction through the module, relative to the front I/O connector. This property is only used when the NI.ChannelEnable for this line is set to true. Changes to this property take effect after running the NI.ChannelConfigurationUpdate command."], "Child Tag"="Physical Channel/port1/line4/Properties/NI.Line.Direction", "Item Indent"=3, "Child Only?"=FALSE, "Glyph Index"=9}, {"Left Cell String"="NI.Line.Enable", "Child Text"=["False", "Read/Write", "Bool", "", "", "", "[0].RW.Bool.port1/line4.NI.Line.Enable", "DIO line output enable", "DIO output enable for one line. When a line is enabled, the input and output buffers for the front I/O connector and the rear I/O connector of the line are configured based on the NI.Line.Direction property. When a line is not enabled, the buffers for both the front I/O connector and the rear I/O connector are configured as inputs. Changes to this property take effect after running the NI.ChannelConfigurationUpdate command."], "Child Tag"="Physical Channel/port1/line4/Properties/NI.Line.Enable", "Item Indent"=3, "Child Only?"=FALSE, "Glyph Index"=9}, {"Left Cell String"="SLSC-12001-030EE1BC-Mod8/port1/line5", "Child Text"=[], "Child Tag"="Physical Channel/port1/line5", "Item Indent"=1, "Child Only?"=FALSE, "Glyph Index"=31}, {"Left Cell String"="Commands", "Child Text"=[], "Child Tag"="Physical Channel/port1/line5/Commands", "Item Indent"=2, "Child Only?"=FALSE, "Glyph Index"=35}, {"Left Cell String"="Properties", "Child Text"=[], "Child Tag"="Physical Channel/port1/line5/Properties", "Item Indent"=2, "Child Only?"=FALSE, "Glyph Index"=36}, {"Left Cell String"="NI.Line.Index", "Child Text"=["D", "Read Only", "U32", "", "", "", "[13].R.U32.port1/line5.NI.Line.Index", "Overall index of this DIO line in the module", "This is the index of this DIO line for the aggregate module properties: NI.FrontInputBufferState, NI.RearInputBufferState, and NI.TestModeValue."], "Child Tag"="Physical Channel/port1/line5/Properties/NI.Line.Index", "Item Indent"=3, "Child Only?"=FALSE, "Glyph Index"=8}, {"Left Cell String"="NI.Line.Direction", "Child Text"=["[0]Input", "Read/Write", "I32", "Enum", "NI.Line.Direction", "[0]Input;[1]Output_Source;[2]Output_Sink;[3]Output_PushPull;", "[0].RW.I32.port1/line5.NI.Line.Direction", "DIO line direction", "Line signal flow direction through the module, relative to the front I/O connector. This property is only used when the NI.ChannelEnable for this line is set to true. Changes to this property take effect after running the NI.ChannelConfigurationUpdate command."], "Child Tag"="Physical Channel/port1/line5/Properties/NI.Line.Direction", "Item Indent"=3, "Child Only?"=FALSE, "Glyph Index"=9}, {"Left Cell String"="NI.Line.Enable", "Child Text"=["False", "Read/Write", "Bool", "", "", "", "[0].RW.Bool.port1/line5.NI.Line.Enable", "DIO line output enable", "DIO output enable for one line. When a line is enabled, the input and output buffers for the front I/O connector and the rear I/O connector of the line are configured based on the NI.Line.Direction property. When a line is not enabled, the buffers for both the front I/O connector and the rear I/O connector are configured as inputs. Changes to this property take effect after running the NI.ChannelConfigurationUpdate command."], "Child Tag"="Physical Channel/port1/line5/Properties/NI.Line.Enable", "Item Indent"=3, "Child Only?"=FALSE, "Glyph Index"=9}, {"Left Cell String"="SLSC-12001-030EE1BC-Mod8/port1/line6", "Child Text"=[], "Child Tag"="Physical Channel/port1/line6", "Item Indent"=1, "Child Only?"=FALSE, "Glyph Index"=31}, {"Left Cell String"="Commands", "Child Text"=[], "Child Tag"="Physical Channel/port1/line6/Commands", "Item Indent"=2, "Child Only?"=FALSE, "Glyph Index"=35}, {"Left Cell String"="Properties", "Child Text"=[], "Child Tag"="Physical Channel/port1/line6/Properties", "Item Indent"=2, "Child Only?"=FALSE, "Glyph Index"=36}, {"Left Cell String"="NI.Line.Index", "Child Text"=["E", "Read Only", "U32", "", "", "", "[14].R.U32.port1/line6.NI.Line.Index", "Overall index of this DIO line in the module", "This is the index of this DIO line for the aggregate module properties: NI.FrontInputBufferState, NI.RearInputBufferState, and NI.TestModeValue."], "Child Tag"="Physical Channel/port1/line6/Properties/NI.Line.Index", "Item Indent"=3, "Child Only?"=FALSE, "Glyph Index"=8}, {"Left Cell String"="NI.Line.Direction", "Child Text"=["[0]Input", "Read/Write", "I32", "Enum", "NI.Line.Direction", "[0]Input;[1]Output_Source;[2]Output_Sink;[3]Output_PushPull;", "[0].RW.I32.port1/line6.NI.Line.Direction", "DIO line direction", "Line signal flow direction through the module, relative to the front I/O connector. This property is only used when the NI.ChannelEnable for this line is set to true. Changes to this property take effect after running the NI.ChannelConfigurationUpdate command."], "Child Tag"="Physical Channel/port1/line6/Properties/NI.Line.Direction", "Item Indent"=3, "Child Only?"=FALSE, "Glyph Index"=9}, {"Left Cell String"="NI.Line.Enable", "Child Text"=["False", "Read/Write", "Bool", "", "", "", "[0].RW.Bool.port1/line6.NI.Line.Enable", "DIO line output enable", "DIO output enable for one line. When a line is enabled, the input and output buffers for the front I/O connector and the rear I/O connector of the line are configured based on the NI.Line.Direction property. When a line is not enabled, the buffers for both the front I/O connector and the rear I/O connector are configured as inputs. Changes to this property take effect after running the NI.ChannelConfigurationUpdate command."], "Child Tag"="Physical Channel/port1/line6/Properties/NI.Line.Enable", "Item Indent"=3, "Child Only?"=FALSE, "Glyph Index"=9}, {"Left Cell String"="SLSC-12001-030EE1BC-Mod8/port1/line7", "Child Text"=[], "Child Tag"="Physical Channel/port1/line7", "Item Indent"=1, "Child Only?"=FALSE, "Glyph Index"=31}, {"Left Cell String"="Commands", "Child Text"=[], "Child Tag"="Physical Channel/port1/line7/Commands", "Item Indent"=2, "Child Only?"=FALSE, "Glyph Index"=35}, {"Left Cell String"="Properties", "Child Text"=[], "Child Tag"="Physical Channel/port1/line7/Properties", "Item Indent"=2, "Child Only?"=FALSE, "Glyph Index"=36}, {"Left Cell String"="NI.Line.Index", "Child Text"=["F", "Read Only", "U32", "", "", "", "[15].R.U32.port1/line7.NI.Line.Index", "Overall index of this DIO line in the module", "This is the index of this DIO line for the aggregate module properties: NI.FrontInputBufferState, NI.RearInputBufferState, and NI.TestModeValue."], "Child Tag"="Physical Channel/port1/line7/Properties/NI.Line.Index", "Item Indent"=3, "Child Only?"=FALSE, "Glyph Index"=8}, {"Left Cell String"="NI.Line.Direction", "Child Text"=["[0]Input", "Read/Write", "I32", "Enum", "NI.Line.Direction", "[0]Input;[1]Output_Source;[2]Output_Sink;[3]Output_PushPull;", "[0].RW.I32.port1/line7.NI.Line.Direction", "DIO line direction", "Line signal flow direction through the module, relative to the front I/O connector. This property is only used when the NI.ChannelEnable for this line is set to true. Changes to this property take effect after running the NI.ChannelConfigurationUpdate command."], "Child Tag"="Physical Channel/port1/line7/Properties/NI.Line.Direction", "Item Indent"=3, "Child Only?"=FALSE, "Glyph Index"=9}, {"Left Cell String"="NI.Line.Enable", "Child Text"=["False", "Read/Write", "Bool", "", "", "", "[0].RW.Bool.port1/line7.NI.Line.Enable", "DIO line output enable", "DIO output enable for one line. When a line is enabled, the input and output buffers for the front I/O connector and the rear I/O connector of the line are configured based on the NI.Line.Direction property. When a line is not enabled, the buffers for both the front I/O connector and the rear I/O connector are configured as inputs. Changes to this property take effect after running the NI.ChannelConfigurationUpdate command."], "Child Tag"="Physical Channel/port1/line7/Properties/NI.Line.Enable", "Item Indent"=3, "Child Only?"=FALSE, "Glyph Index"=9}, {"Left Cell String"="SLSC-12001-030EE1BC-Mod8/port2/line0", "Child Text"=[], "Child Tag"="Physical Channel/port2/line0", "Item Indent"=1, "Child Only?"=FALSE, "Glyph Index"=31}, {"Left Cell String"="Commands", "Child Text"=[], "Child Tag"="Physical Channel/port2/line0/Commands", "Item Indent"=2, "Child Only?"=FALSE, "Glyph Index"=35}, {"Left Cell String"="Properties", "Child Text"=[], "Child Tag"="Physical Channel/port2/line0/Properties", "Item Indent"=2, "Child Only?"=FALSE, "Glyph Index"=36}, {"Left Cell String"="NI.Line.Index", "Child Text"=["10", "Read Only", "U32", "", "", "", "[16].R.U32.port2/line0.NI.Line.Index", "Overall index of this DIO line in the module", "This is the index of this DIO line for the aggregate module properties: NI.FrontInputBufferState, NI.RearInputBufferState, and NI.TestModeValue."], "Child Tag"="Physical Channel/port2/line0/Properties/NI.Line.Index", "Item Indent"=3, "Child Only?"=FALSE, "Glyph Index"=8}, {"Left Cell String"="NI.Line.Direction", "Child Text"=["[0]Input", "Read/Write", "I32", "Enum", "NI.Line.Direction", "[0]Input;[1]Output_Source;[2]Output_Sink;[3]Output_PushPull;", "[0].RW.I32.port2/line0.NI.Line.Direction", "DIO line direction", "Line signal flow direction through the module, relative to the front I/O connector. This property is only used when the NI.ChannelEnable for this line is set to true. Changes to this property take effect after running the NI.ChannelConfigurationUpdate command."], "Child Tag"="Physical Channel/port2/line0/Properties/NI.Line.Direction", "Item Indent"=3, "Child Only?"=FALSE, "Glyph Index"=9}, {"Left Cell String"="NI.Line.Enable", "Child Text"=["False", "Read/Write", "Bool", "", "", "", "[0].RW.Bool.port2/line0.NI.Line.Enable", "DIO line output enable", "DIO output enable for one line. When a line is enabled, the input and output buffers for the front I/O connector and the rear I/O connector of the line are configured based on the NI.Line.Direction property. When a line is not enabled, the buffers for both the front I/O connector and the rear I/O connector are configured as inputs. Changes to this property take effect after running the NI.ChannelConfigurationUpdate command."], "Child Tag"="Physical Channel/port2/line0/Properties/NI.Line.Enable", "Item Indent"=3, "Child Only?"=FALSE, "Glyph Index"=9}, {"Left Cell String"="SLSC-12001-030EE1BC-Mod8/port2/line1", "Child Text"=[], "Child Tag"="Physical Channel/port2/line1", "Item Indent"=1, "Child Only?"=FALSE, "Glyph Index"=31}, {"Left Cell String"="Commands", "Child Text"=[], "Child Tag"="Physical Channel/port2/line1/Commands", "Item Indent"=2, "Child Only?"=FALSE, "Glyph Index"=35}, {"Left Cell String"="Properties", "Child Text"=[], "Child Tag"="Physical Channel/port2/line1/Properties", "Item Indent"=2, "Child Only?"=FALSE, "Glyph Index"=36}, {"Left Cell String"="NI.Line.Index", "Child Text"=["11", "Read Only", "U32", "", "", "", "[17].R.U32.port2/line1.NI.Line.Index", "Overall index of this DIO line in the module", "This is the index of this DIO line for the aggregate module properties: NI.FrontInputBufferState, NI.RearInputBufferState, and NI.TestModeValue."], "Child Tag"="Physical Channel/port2/line1/Properties/NI.Line.Index", "Item Indent"=3, "Child Only?"=FALSE, "Glyph Index"=8}, {"Left Cell String"="NI.Line.Direction", "Child Text"=["[0]Input", "Read/Write", "I32", "Enum", "NI.Line.Direction", "[0]Input;[1]Output_Source;[2]Output_Sink;[3]Output_PushPull;", "[0].RW.I32.port2/line1.NI.Line.Direction", "DIO line direction", "Line signal flow direction through the module, relative to the front I/O connector. This property is only used when the NI.ChannelEnable for this line is set to true. Changes to this property take effect after running the NI.ChannelConfigurationUpdate command."], "Child Tag"="Physical Channel/port2/line1/Properties/NI.Line.Direction", "Item Indent"=3, "Child Only?"=FALSE, "Glyph Index"=9}, {"Left Cell String"="NI.Line.Enable", "Child Text"=["False", "Read/Write", "Bool", "", "", "", "[0].RW.Bool.port2/line1.NI.Line.Enable", "DIO line output enable", "DIO output enable for one line. When a line is enabled, the input and output buffers for the front I/O connector and the rear I/O connector of the line are configured based on the NI.Line.Direction property. When a line is not enabled, the buffers for both the front I/O connector and the rear I/O connector are configured as inputs. Changes to this property take effect after running the NI.ChannelConfigurationUpdate command."], "Child Tag"="Physical Channel/port2/line1/Properties/NI.Line.Enable", "Item Indent"=3, "Child Only?"=FALSE, "Glyph Index"=9}, {"Left Cell String"="SLSC-12001-030EE1BC-Mod8/port2/line2", "Child Text"=[], "Child Tag"="Physical Channel/port2/line2", "Item Indent"=1, "Child Only?"=FALSE, "Glyph Index"=31}, {"Left Cell String"="Commands", "Child Text"=[], "Child Tag"="Physical Channel/port2/line2/Commands", "Item Indent"=2, "Child Only?"=FALSE, "Glyph Index"=35}, {"Left Cell String"="Properties", "Child Text"=[], "Child Tag"="Physical Channel/port2/line2/Properties", "Item Indent"=2, "Child Only?"=FALSE, "Glyph Index"=36}, {"Left Cell String"="NI.Line.Index", "Child Text"=["12", "Read Only", "U32", "", "", "", "[18].R.U32.port2/line2.NI.Line.Index", "Overall index of this DIO line in the module", "This is the index of this DIO line for the aggregate module properties: NI.FrontInputBufferState, NI.RearInputBufferState, and NI.TestModeValue."], "Child Tag"="Physical Channel/port2/line2/Properties/NI.Line.Index", "Item Indent"=3, "Child Only?"=FALSE, "Glyph Index"=8}, {"Left Cell String"="NI.Line.Direction", "Child Text"=["[0]Input", "Read/Write", "I32", "Enum", "NI.Line.Direction", "[0]Input;[1]Output_Source;[2]Output_Sink;[3]Output_PushPull;", "[0].RW.I32.port2/line2.NI.Line.Direction", "DIO line direction", "Line signal flow direction through the module, relative to the front I/O connector. This property is only used when the NI.ChannelEnable for this line is set to true. Changes to this property take effect after running the NI.ChannelConfigurationUpdate command."], "Child Tag"="Physical Channel/port2/line2/Properties/NI.Line.Direction", "Item Indent"=3, "Child Only?"=FALSE, "Glyph Index"=9}, {"Left Cell String"="NI.Line.Enable", "Child Text"=["False", "Read/Write", "Bool", "", "", "", "[0].RW.Bool.port2/line2.NI.Line.Enable", "DIO line output enable", "DIO output enable for one line. When a line is enabled, the input and output buffers for the front I/O connector and the rear I/O connector of the line are configured based on the NI.Line.Direction property. When a line is not enabled, the buffers for both the front I/O connector and the rear I/O connector are configured as inputs. Changes to this property take effect after running the NI.ChannelConfigurationUpdate command."], "Child Tag"="Physical Channel/port2/line2/Properties/NI.Line.Enable", "Item Indent"=3, "Child Only?"=FALSE, "Glyph Index"=9}, {"Left Cell String"="SLSC-12001-030EE1BC-Mod8/port2/line3", "Child Text"=[], "Child Tag"="Physical Channel/port2/line3", "Item Indent"=1, "Child Only?"=FALSE, "Glyph Index"=31}, {"Left Cell String"="Commands", "Child Text"=[], "Child Tag"="Physical Channel/port2/line3/Commands", "Item Indent"=2, "Child Only?"=FALSE, "Glyph Index"=35}, {"Left Cell String"="Properties", "Child Text"=[], "Child Tag"="Physical Channel/port2/line3/Properties", "Item Indent"=2, "Child Only?"=FALSE, "Glyph Index"=36}, {"Left Cell String"="NI.Line.Index", "Child Text"=["13", "Read Only", "U32", "", "", "", "[19].R.U32.port2/line3.NI.Line.Index", "Overall index of this DIO line in the module", "This is the index of this DIO line for the aggregate module properties: NI.FrontInputBufferState, NI.RearInputBufferState, and NI.TestModeValue."], "Child Tag"="Physical Channel/port2/line3/Properties/NI.Line.Index", "Item Indent"=3, "Child Only?"=FALSE, "Glyph Index"=8}, {"Left Cell String"="NI.Line.Direction", "Child Text"=["[0]Input", "Read/Write", "I32", "Enum", "NI.Line.Direction", "[0]Input;[1]Output_Source;[2]Output_Sink;[3]Output_PushPull;", "[0].RW.I32.port2/line3.NI.Line.Direction", "DIO line direction", "Line signal flow direction through the module, relative to the front I/O connector. This property is only used when the NI.ChannelEnable for this line is set to true. Changes to this property take effect after running the NI.ChannelConfigurationUpdate command."], "Child Tag"="Physical Channel/port2/line3/Properties/NI.Line.Direction", "Item Indent"=3, "Child Only?"=FALSE, "Glyph Index"=9}, {"Left Cell String"="NI.Line.Enable", "Child Text"=["False", "Read/Write", "Bool", "", "", "", "[0].RW.Bool.port2/line3.NI.Line.Enable", "DIO line output enable", "DIO output enable for one line. When a line is enabled, the input and output buffers for the front I/O connector and the rear I/O connector of the line are configured based on the NI.Line.Direction property. When a line is not enabled, the buffers for both the front I/O connector and the rear I/O connector are configured as inputs. Changes to this property take effect after running the NI.ChannelConfigurationUpdate command."], "Child Tag"="Physical Channel/port2/line3/Properties/NI.Line.Enable", "Item Indent"=3, "Child Only?"=FALSE, "Glyph Index"=9}, {"Left Cell String"="SLSC-12001-030EE1BC-Mod8/port2/line4", "Child Text"=[], "Child Tag"="Physical Channel/port2/line4", "Item Indent"=1, "Child Only?"=FALSE, "Glyph Index"=31}, {"Left Cell String"="Commands", "Child Text"=[], "Child Tag"="Physical Channel/port2/line4/Commands", "Item Indent"=2, "Child Only?"=FALSE, "Glyph Index"=35}, {"Left Cell String"="Properties", "Child Text"=[], "Child Tag"="Physical Channel/port2/line4/Properties", "Item Indent"=2, "Child Only?"=FALSE, "Glyph Index"=36}, {"Left Cell String"="NI.Line.Index", "Child Text"=["14", "Read Only", "U32", "", "", "", "[20].R.U32.port2/line4.NI.Line.Index", "Overall index of this DIO line in the module", "This is the index of this DIO line for the aggregate module properties: NI.FrontInputBufferState, NI.RearInputBufferState, and NI.TestModeValue."], "Child Tag"="Physical Channel/port2/line4/Properties/NI.Line.Index", "Item Indent"=3, "Child Only?"=FALSE, "Glyph Index"=8}, {"Left Cell String"="NI.Line.Direction", "Child Text"=["[0]Input", "Read/Write", "I32", "Enum", "NI.Line.Direction", "[0]Input;[1]Output_Source;[2]Output_Sink;[3]Output_PushPull;", "[0].RW.I32.port2/line4.NI.Line.Direction", "DIO line direction", "Line signal flow direction through the module, relative to the front I/O connector. This property is only used when the NI.ChannelEnable for this line is set to true. Changes to this property take effect after running the NI.ChannelConfigurationUpdate command."], "Child Tag"="Physical Channel/port2/line4/Properties/NI.Line.Direction", "Item Indent"=3, "Child Only?"=FALSE, "Glyph Index"=9}, {"Left Cell String"="NI.Line.Enable", "Child Text"=["False", "Read/Write", "Bool", "", "", "", "[0].RW.Bool.port2/line4.NI.Line.Enable", "DIO line output enable", "DIO output enable for one line. When a line is enabled, the input and output buffers for the front I/O connector and the rear I/O connector of the line are configured based on the NI.Line.Direction property. When a line is not enabled, the buffers for both the front I/O connector and the rear I/O connector are configured as inputs. Changes to this property take effect after running the NI.ChannelConfigurationUpdate command."], "Child Tag"="Physical Channel/port2/line4/Properties/NI.Line.Enable", "Item Indent"=3, "Child Only?"=FALSE, "Glyph Index"=9}, {"Left Cell String"="SLSC-12001-030EE1BC-Mod8/port2/line5", "Child Text"=[], "Child Tag"="Physical Channel/port2/line5", "Item Indent"=1, "Child Only?"=FALSE, "Glyph Index"=31}, {"Left Cell String"="Commands", "Child Text"=[], "Child Tag"="Physical Channel/port2/line5/Commands", "Item Indent"=2, "Child Only?"=FALSE, "Glyph Index"=35}, {"Left Cell String"="Properties", "Child Text"=[], "Child Tag"="Physical Channel/port2/line5/Properties", "Item Indent"=2, "Child Only?"=FALSE, "Glyph Index"=36}, {"Left Cell String"="NI.Line.Index", "Child Text"=["15", "Read Only", "U32", "", "", "", "[21].R.U32.port2/line5.NI.Line.Index", "Overall index of this DIO line in the module", "This is the index of this DIO line for the aggregate module properties: NI.FrontInputBufferState, NI.RearInputBufferState, and NI.TestModeValue."], "Child Tag"="Physical Channel/port2/line5/Properties/NI.Line.Index", "Item Indent"=3, "Child Only?"=FALSE, "Glyph Index"=8}, {"Left Cell String"="NI.Line.Direction", "Child Text"=["[0]Input", "Read/Write", "I32", "Enum", "NI.Line.Direction", "[0]Input;[1]Output_Source;[2]Output_Sink;[3]Output_PushPull;", "[0].RW.I32.port2/line5.NI.Line.Direction", "DIO line direction", "Line signal flow direction through the module, relative to the front I/O connector. This property is only used when the NI.ChannelEnable for this line is set to true. Changes to this property take effect after running the NI.ChannelConfigurationUpdate command."], "Child Tag"="Physical Channel/port2/line5/Properties/NI.Line.Direction", "Item Indent"=3, "Child Only?"=FALSE, "Glyph Index"=9}, {"Left Cell String"="NI.Line.Enable", "Child Text"=["False", "Read/Write", "Bool", "", "", "", "[0].RW.Bool.port2/line5.NI.Line.Enable", "DIO line output enable", "DIO output enable for one line. When a line is enabled, the input and output buffers for the front I/O connector and the rear I/O connector of the line are configured based on the NI.Line.Direction property. When a line is not enabled, the buffers for both the front I/O connector and the rear I/O connector are configured as inputs. Changes to this property take effect after running the NI.ChannelConfigurationUpdate command."], "Child Tag"="Physical Channel/port2/line5/Properties/NI.Line.Enable", "Item Indent"=3, "Child Only?"=FALSE, "Glyph Index"=9}, {"Left Cell String"="SLSC-12001-030EE1BC-Mod8/port2/line6", "Child Text"=[], "Child Tag"="Physical Channel/port2/line6", "Item Indent"=1, "Child Only?"=FALSE, "Glyph Index"=31}, {"Left Cell String"="Commands", "Child Text"=[], "Child Tag"="Physical Channel/port2/line6/Commands", "Item Indent"=2, "Child Only?"=FALSE, "Glyph Index"=35}, {"Left Cell String"="Properties", "Child Text"=[], "Child Tag"="Physical Channel/port2/line6/Properties", "Item Indent"=2, "Child Only?"=FALSE, "Glyph Index"=36}, {"Left Cell String"="NI.Line.Index", "Child Text"=["16", "Read Only", "U32", "", "", "", "[22].R.U32.port2/line6.NI.Line.Index", "Overall index of this DIO line in the module", "This is the index of this DIO line for the aggregate module properties: NI.FrontInputBufferState, NI.RearInputBufferState, and NI.TestModeValue."], "Child Tag"="Physical Channel/port2/line6/Properties/NI.Line.Index", "Item Indent"=3, "Child Only?"=FALSE, "Glyph Index"=8}, {"Left Cell String"="NI.Line.Direction", "Child Text"=["[0]Input", "Read/Write", "I32", "Enum", "NI.Line.Direction", "[0]Input;[1]Output_Source;[2]Output_Sink;[3]Output_PushPull;", "[0].RW.I32.port2/line6.NI.Line.Direction", "DIO line direction", "Line signal flow direction through the module, relative to the front I/O connector. This property is only used when the NI.ChannelEnable for this line is set to true. Changes to this property take effect after running the NI.ChannelConfigurationUpdate command."], "Child Tag"="Physical Channel/port2/line6/Properties/NI.Line.Direction", "Item Indent"=3, "Child Only?"=FALSE, "Glyph Index"=9}, {"Left Cell String"="NI.Line.Enable", "Child Text"=["False", "Read/Write", "Bool", "", "", "", "[0].RW.Bool.port2/line6.NI.Line.Enable", "DIO line output enable", "DIO output enable for one line. When a line is enabled, the input and output buffers for the front I/O connector and the rear I/O connector of the line are configured based on the NI.Line.Direction property. When a line is not enabled, the buffers for both the front I/O connector and the rear I/O connector are configured as inputs. Changes to this property take effect after running the NI.ChannelConfigurationUpdate command."], "Child Tag"="Physical Channel/port2/line6/Properties/NI.Line.Enable", "Item Indent"=3, "Child Only?"=FALSE, "Glyph Index"=9}, {"Left Cell String"="SLSC-12001-030EE1BC-Mod8/port2/line7", "Child Text"=[], "Child Tag"="Physical Channel/port2/line7", "Item Indent"=1, "Child Only?"=FALSE, "Glyph Index"=31}, {"Left Cell String"="Commands", "Child Text"=[], "Child Tag"="Physical Channel/port2/line7/Commands", "Item Indent"=2, "Child Only?"=FALSE, "Glyph Index"=35}, {"Left Cell String"="Properties", "Child Text"=[], "Child Tag"="Physical Channel/port2/line7/Properties", "Item Indent"=2, "Child Only?"=FALSE, "Glyph Index"=36}, {"Left Cell String"="NI.Line.Index", "Child Text"=["17", "Read Only", "U32", "", "", "", "[23].R.U32.port2/line7.NI.Line.Index", "Overall index of this DIO line in the module", "This is the index of this DIO line for the aggregate module properties: NI.FrontInputBufferState, NI.RearInputBufferState, and NI.TestModeValue."], "Child Tag"="Physical Channel/port2/line7/Properties/NI.Line.Index", "Item Indent"=3, "Child Only?"=FALSE, "Glyph Index"=8}, {"Left Cell String"="NI.Line.Direction", "Child Text"=["[0]Input", "Read/Write", "I32", "Enum", "NI.Line.Direction", "[0]Input;[1]Output_Source;[2]Output_Sink;[3]Output_PushPull;", "[0].RW.I32.port2/line7.NI.Line.Direction", "DIO line direction", "Line signal flow direction through the module, relative to the front I/O connector. This property is only used when the NI.ChannelEnable for this line is set to true. Changes to this property take effect after running the NI.ChannelConfigurationUpdate command."], "Child Tag"="Physical Channel/port2/line7/Properties/NI.Line.Direction", "Item Indent"=3, "Child Only?"=FALSE, "Glyph Index"=9}, {"Left Cell String"="NI.Line.Enable", "Child Text"=["False", "Read/Write", "Bool", "", "", "", "[0].RW.Bool.port2/line7.NI.Line.Enable", "DIO line output enable", "DIO output enable for one line. When a line is enabled, the input and output buffers for the front I/O connector and the rear I/O connector of the line are configured based on the NI.Line.Direction property. When a line is not enabled, the buffers for both the front I/O connector and the rear I/O connector are configured as inputs. Changes to this property take effect after running the NI.ChannelConfigurationUpdate command."], "Child Tag"="Physical Channel/port2/line7/Properties/NI.Line.Enable", "Item Indent"=3, "Child Only?"=FALSE, "Glyph Index"=9}, {"Left Cell String"="SLSC-12001-030EE1BC-Mod8/port3/line0", "Child Text"=[], "Child Tag"="Physical Channel/port3/line0", "Item Indent"=1, "Child Only?"=FALSE, "Glyph Index"=31}, {"Left Cell String"="Commands", "Child Text"=[], "Child Tag"="Physical Channel/port3/line0/Commands", "Item Indent"=2, "Child Only?"=FALSE, "Glyph Index"=35}, {"Left Cell String"="Properties", "Child Text"=[], "Child Tag"="Physical Channel/port3/line0/Properties", "Item Indent"=2, "Child Only?"=FALSE, "Glyph Index"=36}, {"Left Cell String"="NI.Line.Index", "Child Text"=["18", "Read Only", "U32", "", "", "", "[24].R.U32.port3/line0.NI.Line.Index", "Overall index of this DIO line in the module", "This is the index of this DIO line for the aggregate module properties: NI.FrontInputBufferState, NI.RearInputBufferState, and NI.TestModeValue."], "Child Tag"="Physical Channel/port3/line0/Properties/NI.Line.Index", "Item Indent"=3, "Child Only?"=FALSE, "Glyph Index"=8}, {"Left Cell String"="NI.Line.Direction", "Child Text"=["[0]Input", "Read/Write", "I32", "Enum", "NI.Line.Direction", "[0]Input;[1]Output_Source;[2]Output_Sink;[3]Output_PushPull;", "[0].RW.I32.port3/line0.NI.Line.Direction", "DIO line direction", "Line signal flow direction through the module, relative to the front I/O connector. This property is only used when the NI.ChannelEnable for this line is set to true. Changes to this property take effect after running the NI.ChannelConfigurationUpdate command."], "Child Tag"="Physical Channel/port3/line0/Properties/NI.Line.Direction", "Item Indent"=3, "Child Only?"=FALSE, "Glyph Index"=9}, {"Left Cell String"="NI.Line.Enable", "Child Text"=["False", "Read/Write", "Bool", "", "", "", "[0].RW.Bool.port3/line0.NI.Line.Enable", "DIO line output enable", "DIO output enable for one line. When a line is enabled, the input and output buffers for the front I/O connector and the rear I/O connector of the line are configured based on the NI.Line.Direction property. When a line is not enabled, the buffers for both the front I/O connector and the rear I/O connector are configured as inputs. Changes to this property take effect after running the NI.ChannelConfigurationUpdate command."], "Child Tag"="Physical Channel/port3/line0/Properties/NI.Line.Enable", "Item Indent"=3, "Child Only?"=FALSE, "Glyph Index"=9}, {"Left Cell String"="SLSC-12001-030EE1BC-Mod8/port3/line1", "Child Text"=[], "Child Tag"="Physical Channel/port3/line1", "Item Indent"=1, "Child Only?"=FALSE, "Glyph Index"=31}, {"Left Cell String"="Commands", "Child Text"=[], "Child Tag"="Physical Channel/port3/line1/Commands", "Item Indent"=2, "Child Only?"=FALSE, "Glyph Index"=35}, {"Left Cell String"="Properties", "Child Text"=[], "Child Tag"="Physical Channel/port3/line1/Properties", "Item Indent"=2, "Child Only?"=FALSE, "Glyph Index"=36}, {"Left Cell String"="NI.Line.Index", "Child Text"=["19", "Read Only", "U32", "", "", "", "[25].R.U32.port3/line1.NI.Line.Index", "Overall index of this DIO line in the module", "This is the index of this DIO line for the aggregate module properties: NI.FrontInputBufferState, NI.RearInputBufferState, and NI.TestModeValue."], "Child Tag"="Physical Channel/port3/line1/Properties/NI.Line.Index", "Item Indent"=3, "Child Only?"=FALSE, "Glyph Index"=8}, {"Left Cell String"="NI.Line.Direction", "Child Text"=["[0]Input", "Read/Write", "I32", "Enum", "NI.Line.Direction", "[0]Input;[1]Output_Source;[2]Output_Sink;[3]Output_PushPull;", "[0].RW.I32.port3/line1.NI.Line.Direction", "DIO line direction", "Line signal flow direction through the module, relative to the front I/O connector. This property is only used when the NI.ChannelEnable for this line is set to true. Changes to this property take effect after running the NI.ChannelConfigurationUpdate command."], "Child Tag"="Physical Channel/port3/line1/Properties/NI.Line.Direction", "Item Indent"=3, "Child Only?"=FALSE, "Glyph Index"=9}, {"Left Cell String"="NI.Line.Enable", "Child Text"=["False", "Read/Write", "Bool", "", "", "", "[0].RW.Bool.port3/line1.NI.Line.Enable", "DIO line output enable", "DIO output enable for one line. When a line is enabled, the input and output buffers for the front I/O connector and the rear I/O connector of the line are configured based on the NI.Line.Direction property. When a line is not enabled, the buffers for both the front I/O connector and the rear I/O connector are configured as inputs. Changes to this property take effect after running the NI.ChannelConfigurationUpdate command."], "Child Tag"="Physical Channel/port3/line1/Properties/NI.Line.Enable", "Item Indent"=3, "Child Only?"=FALSE, "Glyph Index"=9}, {"Left Cell String"="SLSC-12001-030EE1BC-Mod8/port3/line2", "Child Text"=[], "Child Tag"="Physical Channel/port3/line2", "Item Indent"=1, "Child Only?"=FALSE, "Glyph Index"=31}, {"Left Cell String"="Commands", "Child Text"=[], "Child Tag"="Physical Channel/port3/line2/Commands", "Item Indent"=2, "Child Only?"=FALSE, "Glyph Index"=35}, {"Left Cell String"="Properties", "Child Text"=[], "Child Tag"="Physical Channel/port3/line2/Properties", "Item Indent"=2, "Child Only?"=FALSE, "Glyph Index"=36}, {"Left Cell String"="NI.Line.Index", "Child Text"=["1A", "Read Only", "U32", "", "", "", "[26].R.U32.port3/line2.NI.Line.Index", "Overall index of this DIO line in the module", "This is the index of this DIO line for the aggregate module properties: NI.FrontInputBufferState, NI.RearInputBufferState, and NI.TestModeValue."], "Child Tag"="Physical Channel/port3/line2/Properties/NI.Line.Index", "Item Indent"=3, "Child Only?"=FALSE, "Glyph Index"=8}, {"Left Cell String"="NI.Line.Direction", "Child Text"=["[0]Input", "Read/Write", "I32", "Enum", "NI.Line.Direction", "[0]Input;[1]Output_Source;[2]Output_Sink;[3]Output_PushPull;", "[0].RW.I32.port3/line2.NI.Line.Direction", "DIO line direction", "Line signal flow direction through the module, relative to the front I/O connector. This property is only used when the NI.ChannelEnable for this line is set to true. Changes to this property take effect after running the NI.ChannelConfigurationUpdate command."], "Child Tag"="Physical Channel/port3/line2/Properties/NI.Line.Direction", "Item Indent"=3, "Child Only?"=FALSE, "Glyph Index"=9}, {"Left Cell String"="NI.Line.Enable", "Child Text"=["False", "Read/Write", "Bool", "", "", "", "[0].RW.Bool.port3/line2.NI.Line.Enable", "DIO line output enable", "DIO output enable for one line. When a line is enabled, the input and output buffers for the front I/O connector and the rear I/O connector of the line are configured based on the NI.Line.Direction property. When a line is not enabled, the buffers for both the front I/O connector and the rear I/O connector are configured as inputs. Changes to this property take effect after running the NI.ChannelConfigurationUpdate command."], "Child Tag"="Physical Channel/port3/line2/Properties/NI.Line.Enable", "Item Indent"=3, "Child Only?"=FALSE, "Glyph Index"=9}, {"Left Cell String"="SLSC-12001-030EE1BC-Mod8/port3/line3", "Child Text"=[], "Child Tag"="Physical Channel/port3/line3", "Item Indent"=1, "Child Only?"=FALSE, "Glyph Index"=31}, {"Left Cell String"="Commands", "Child Text"=[], "Child Tag"="Physical Channel/port3/line3/Commands", "Item Indent"=2, "Child Only?"=FALSE, "Glyph Index"=35}, {"Left Cell String"="Properties", "Child Text"=[], "Child Tag"="Physical Channel/port3/line3/Properties", "Item Indent"=2, "Child Only?"=FALSE, "Glyph Index"=36}, {"Left Cell String"="NI.Line.Index", "Child Text"=["1B", "Read Only", "U32", "", "", "", "[27].R.U32.port3/line3.NI.Line.Index", "Overall index of this DIO line in the module", "This is the index of this DIO line for the aggregate module properties: NI.FrontInputBufferState, NI.RearInputBufferState, and NI.TestModeValue."], "Child Tag"="Physical Channel/port3/line3/Properties/NI.Line.Index", "Item Indent"=3, "Child Only?"=FALSE, "Glyph Index"=8}, {"Left Cell String"="NI.Line.Direction", "Child Text"=["[0]Input", "Read/Write", "I32", "Enum", "NI.Line.Direction", "[0]Input;[1]Output_Source;[2]Output_Sink;[3]Output_PushPull;", "[0].RW.I32.port3/line3.NI.Line.Direction", "DIO line direction", "Line signal flow direction through the module, relative to the front I/O connector. This property is only used when the NI.ChannelEnable for this line is set to true. Changes to this property take effect after running the NI.ChannelConfigurationUpdate command."], "Child Tag"="Physical Channel/port3/line3/Properties/NI.Line.Direction", "Item Indent"=3, "Child Only?"=FALSE, "Glyph Index"=9}, {"Left Cell String"="NI.Line.Enable", "Child Text"=["False", "Read/Write", "Bool", "", "", "", "[0].RW.Bool.port3/line3.NI.Line.Enable", "DIO line output enable", "DIO output enable for one line. When a line is enabled, the input and output buffers for the front I/O connector and the rear I/O connector of the line are configured based on the NI.Line.Direction property. When a line is not enabled, the buffers for both the front I/O connector and the rear I/O connector are configured as inputs. Changes to this property take effect after running the NI.ChannelConfigurationUpdate command."], "Child Tag"="Physical Channel/port3/line3/Properties/NI.Line.Enable", "Item Indent"=3, "Child Only?"=FALSE, "Glyph Index"=9}, {"Left Cell String"="SLSC-12001-030EE1BC-Mod8/port3/line4", "Child Text"=[], "Child Tag"="Physical Channel/port3/line4", "Item Indent"=1, "Child Only?"=FALSE, "Glyph Index"=31}, {"Left Cell String"="Commands", "Child Text"=[], "Child Tag"="Physical Channel/port3/line4/Commands", "Item Indent"=2, "Child Only?"=FALSE, "Glyph Index"=35}, {"Left Cell String"="Properties", "Child Text"=[], "Child Tag"="Physical Channel/port3/line4/Properties", "Item Indent"=2, "Child Only?"=FALSE, "Glyph Index"=36}, {"Left Cell String"="NI.Line.Index", "Child Text"=["1C", "Read Only", "U32", "", "", "", "[28].R.U32.port3/line4.NI.Line.Index", "Overall index of this DIO line in the module", "This is the index of this DIO line for the aggregate module properties: NI.FrontInputBufferState, NI.RearInputBufferState, and NI.TestModeValue."], "Child Tag"="Physical Channel/port3/line4/Properties/NI.Line.Index", "Item Indent"=3, "Child Only?"=FALSE, "Glyph Index"=8}, {"Left Cell String"="NI.Line.Direction", "Child Text"=["[0]Input", "Read/Write", "I32", "Enum", "NI.Line.Direction", "[0]Input;[1]Output_Source;[2]Output_Sink;[3]Output_PushPull;", "[0].RW.I32.port3/line4.NI.Line.Direction", "DIO line direction", "Line signal flow direction through the module, relative to the front I/O connector. This property is only used when the NI.ChannelEnable for this line is set to true. Changes to this property take effect after running the NI.ChannelConfigurationUpdate command."], "Child Tag"="Physical Channel/port3/line4/Properties/NI.Line.Direction", "Item Indent"=3, "Child Only?"=FALSE, "Glyph Index"=9}, {"Left Cell String"="NI.Line.Enable", "Child Text"=["False", "Read/Write", "Bool", "", "", "", "[0].RW.Bool.port3/line4.NI.Line.Enable", "DIO line output enable", "DIO output enable for one line. When a line is enabled, the input and output buffers for the front I/O connector and the rear I/O connector of the line are configured based on the NI.Line.Direction property. When a line is not enabled, the buffers for both the front I/O connector and the rear I/O connector are configured as inputs. Changes to this property take effect after running the NI.ChannelConfigurationUpdate command."], "Child Tag"="Physical Channel/port3/line4/Properties/NI.Line.Enable", "Item Indent"=3, "Child Only?"=FALSE, "Glyph Index"=9}, {"Left Cell String"="SLSC-12001-030EE1BC-Mod8/port3/line5", "Child Text"=[], "Child Tag"="Physical Channel/port3/line5", "Item Indent"=1, "Child Only?"=FALSE, "Glyph Index"=31}, {"Left Cell String"="Commands", "Child Text"=[], "Child Tag"="Physical Channel/port3/line5/Commands", "Item Indent"=2, "Child Only?"=FALSE, "Glyph Index"=35}, {"Left Cell String"="Properties", "Child Text"=[], "Child Tag"="Physical Channel/port3/line5/Properties", "Item Indent"=2, "Child Only?"=FALSE, "Glyph Index"=36}, {"Left Cell String"="NI.Line.Index", "Child Text"=["1D", "Read Only", "U32", "", "", "", "[29].R.U32.port3/line5.NI.Line.Index", "Overall index of this DIO line in the module", "This is the index of this DIO line for the aggregate module properties: NI.FrontInputBufferState, NI.RearInputBufferState, and NI.TestModeValue."], "Child Tag"="Physical Channel/port3/line5/Properties/NI.Line.Index", "Item Indent"=3, "Child Only?"=FALSE, "Glyph Index"=8}, {"Left Cell String"="NI.Line.Direction", "Child Text"=["[0]Input", "Read/Write", "I32", "Enum", "NI.Line.Direction", "[0]Input;[1]Output_Source;[2]Output_Sink;[3]Output_PushPull;", "[0].RW.I32.port3/line5.NI.Line.Direction", "DIO line direction", "Line signal flow direction through the module, relative to the front I/O connector. This property is only used when the NI.ChannelEnable for this line is set to true. Changes to this property take effect after running the NI.ChannelConfigurationUpdate command."], "Child Tag"="Physical Channel/port3/line5/Properties/NI.Line.Direction", "Item Indent"=3, "Child Only?"=FALSE, "Glyph Index"=9}, {"Left Cell String"="NI.Line.Enable", "Child Text"=["False", "Read/Write", "Bool", "", "", "", "[0].RW.Bool.port3/line5.NI.Line.Enable", "DIO line output enable", "DIO output enable for one line. When a line is enabled, the input and output buffers for the front I/O connector and the rear I/O connector of the line are configured based on the NI.Line.Direction property. When a line is not enabled, the buffers for both the front I/O connector and the rear I/O connector are configured as inputs. Changes to this property take effect after running the NI.ChannelConfigurationUpdate command."], "Child Tag"="Physical Channel/port3/line5/Properties/NI.Line.Enable", "Item Indent"=3, "Child Only?"=FALSE, "Glyph Index"=9}, {"Left Cell String"="SLSC-12001-030EE1BC-Mod8/port3/line6", "Child Text"=[], "Child Tag"="Physical Channel/port3/line6", "Item Indent"=1, "Child Only?"=FALSE, "Glyph Index"=31}, {"Left Cell String"="Commands", "Child Text"=[], "Child Tag"="Physical Channel/port3/line6/Commands", "Item Indent"=2, "Child Only?"=FALSE, "Glyph Index"=35}, {"Left Cell String"="Properties", "Child Text"=[], "Child Tag"="Physical Channel/port3/line6/Properties", "Item Indent"=2, "Child Only?"=FALSE, "Glyph Index"=36}, {"Left Cell String"="NI.Line.Index", "Child Text"=["1E", "Read Only", "U32", "", "", "", "[30].R.U32.port3/line6.NI.Line.Index", "Overall index of this DIO line in the module", "This is the index of this DIO line for the aggregate module properties: NI.FrontInputBufferState, NI.RearInputBufferState, and NI.TestModeValue."], "Child Tag"="Physical Channel/port3/line6/Properties/NI.Line.Index", "Item Indent"=3, "Child Only?"=FALSE, "Glyph Index"=8}, {"Left Cell String"="NI.Line.Direction", "Child Text"=["[0]Input", "Read/Write", "I32", "Enum", "NI.Line.Direction", "[0]Input;[1]Output_Source;[2]Output_Sink;[3]Output_PushPull;", "[0].RW.I32.port3/line6.NI.Line.Direction", "DIO line direction", "Line signal flow direction through the module, relative to the front I/O connector. This property is only used when the NI.ChannelEnable for this line is set to true. Changes to this property take effect after running the NI.ChannelConfigurationUpdate command."], "Child Tag"="Physical Channel/port3/line6/Properties/NI.Line.Direction", "Item Indent"=3, "Child Only?"=FALSE, "Glyph Index"=9}, {"Left Cell String"="NI.Line.Enable", "Child Text"=["False", "Read/Write", "Bool", "", "", "", "[0].RW.Bool.port3/line6.NI.Line.Enable", "DIO line output enable", "DIO output enable for one line. When a line is enabled, the input and output buffers for the front I/O connector and the rear I/O connector of the line are configured based on the NI.Line.Direction property. When a line is not enabled, the buffers for both the front I/O connector and the rear I/O connector are configured as inputs. Changes to this property take effect after running the NI.ChannelConfigurationUpdate command."], "Child Tag"="Physical Channel/port3/line6/Properties/NI.Line.Enable", "Item Indent"=3, "Child Only?"=FALSE, "Glyph Index"=9}, {"Left Cell String"="SLSC-12001-030EE1BC-Mod8/port3/line7", "Child Text"=[], "Child Tag"="Physical Channel/port3/line7", "Item Indent"=1, "Child Only?"=FALSE, "Glyph Index"=31}, {"Left Cell String"="Commands", "Child Text"=[], "Child Tag"="Physical Channel/port3/line7/Commands", "Item Indent"=2, "Child Only?"=FALSE, "Glyph Index"=35}, {"Left Cell String"="Properties", "Child Text"=[], "Child Tag"="Physical Channel/port3/line7/Properties", "Item Indent"=2, "Child Only?"=FALSE, "Glyph Index"=36}, {"Left Cell String"="NI.Line.Index", "Child Text"=["1F", "Read Only", "U32", "", "", "", "[31].R.U32.port3/line7.NI.Line.Index", "Overall index of this DIO line in the module", "This is the index of this DIO line for the aggregate module properties: NI.FrontInputBufferState, NI.RearInputBufferState, and NI.TestModeValue."], "Child Tag"="Physical Channel/port3/line7/Properties/NI.Line.Index", "Item Indent"=3, "Child Only?"=FALSE, "Glyph Index"=8}, {"Left Cell String"="NI.Line.Direction", "Child Text"=["[0]Input", "Read/Write", "I32", "Enum", "NI.Line.Direction", "[0]Input;[1]Output_Source;[2]Output_Sink;[3]Output_PushPull;", "[0].RW.I32.port3/line7.NI.Line.Direction", "DIO line direction", "Line signal flow direction through the module, relative to the front I/O connector. This property is only used when the NI.ChannelEnable for this line is set to true. Changes to this property take effect after running the NI.ChannelConfigurationUpdate command."], "Child Tag"="Physical Channel/port3/line7/Properties/NI.Line.Direction", "Item Indent"=3, "Child Only?"=FALSE, "Glyph Index"=9}, {"Left Cell String"="NI.Line.Enable", "Child Text"=["False", "Read/Write", "Bool", "", "", "", "[0].RW.Bool.port3/line7.NI.Line.Enable", "DIO line output enable", "DIO output enable for one line. When a line is enabled, the input and output buffers for the front I/O connector and the rear I/O connector of the line are configured based on the NI.Line.Direction property. When a line is not enabled, the buffers for both the front I/O connector and the rear I/O connector are configured as inputs. Changes to this property take effect after running the NI.ChannelConfigurationUpdate command."], "Child Tag"="Physical Channel/port3/line7/Properties/NI.Line.Enable", "Item Indent"=3, "Child Only?"=FALSE, "Glyph Index"=9}])   [LabVIEW 2017, in "SLSC Tree Control.lvlib"]
doc: "Creates a SLSC tree control based on the SLSC EDS datatype (Capabilities)."
uses:
  SLSC Tree Control.lvlib
  SLSC EDS API/JSON parsing/EDSjsonStructure.ctl
  SLSC EDS API/JSON parsing/enum.ctl
  SLSC EDS API/JSON parsing/property.ctl
  SLSC EDS API/JSON parsing/command.ctl
  SLSC EDS API/JSON parsing/scale.ctl
  SLSC EDS API/JSON parsing/physicalChannel.ctl
  SLSC EDS API/JSON parsing/register.ctl
panel:
  out "Array 2":string[](array[string])
  out "Array":string[](array[string])
  in  "stop":bool
  out "Property tree 2":string[](array[string])
  in  "Property tree":string[](tree)
  # "not working\nregisterMap->registers->initialValue"
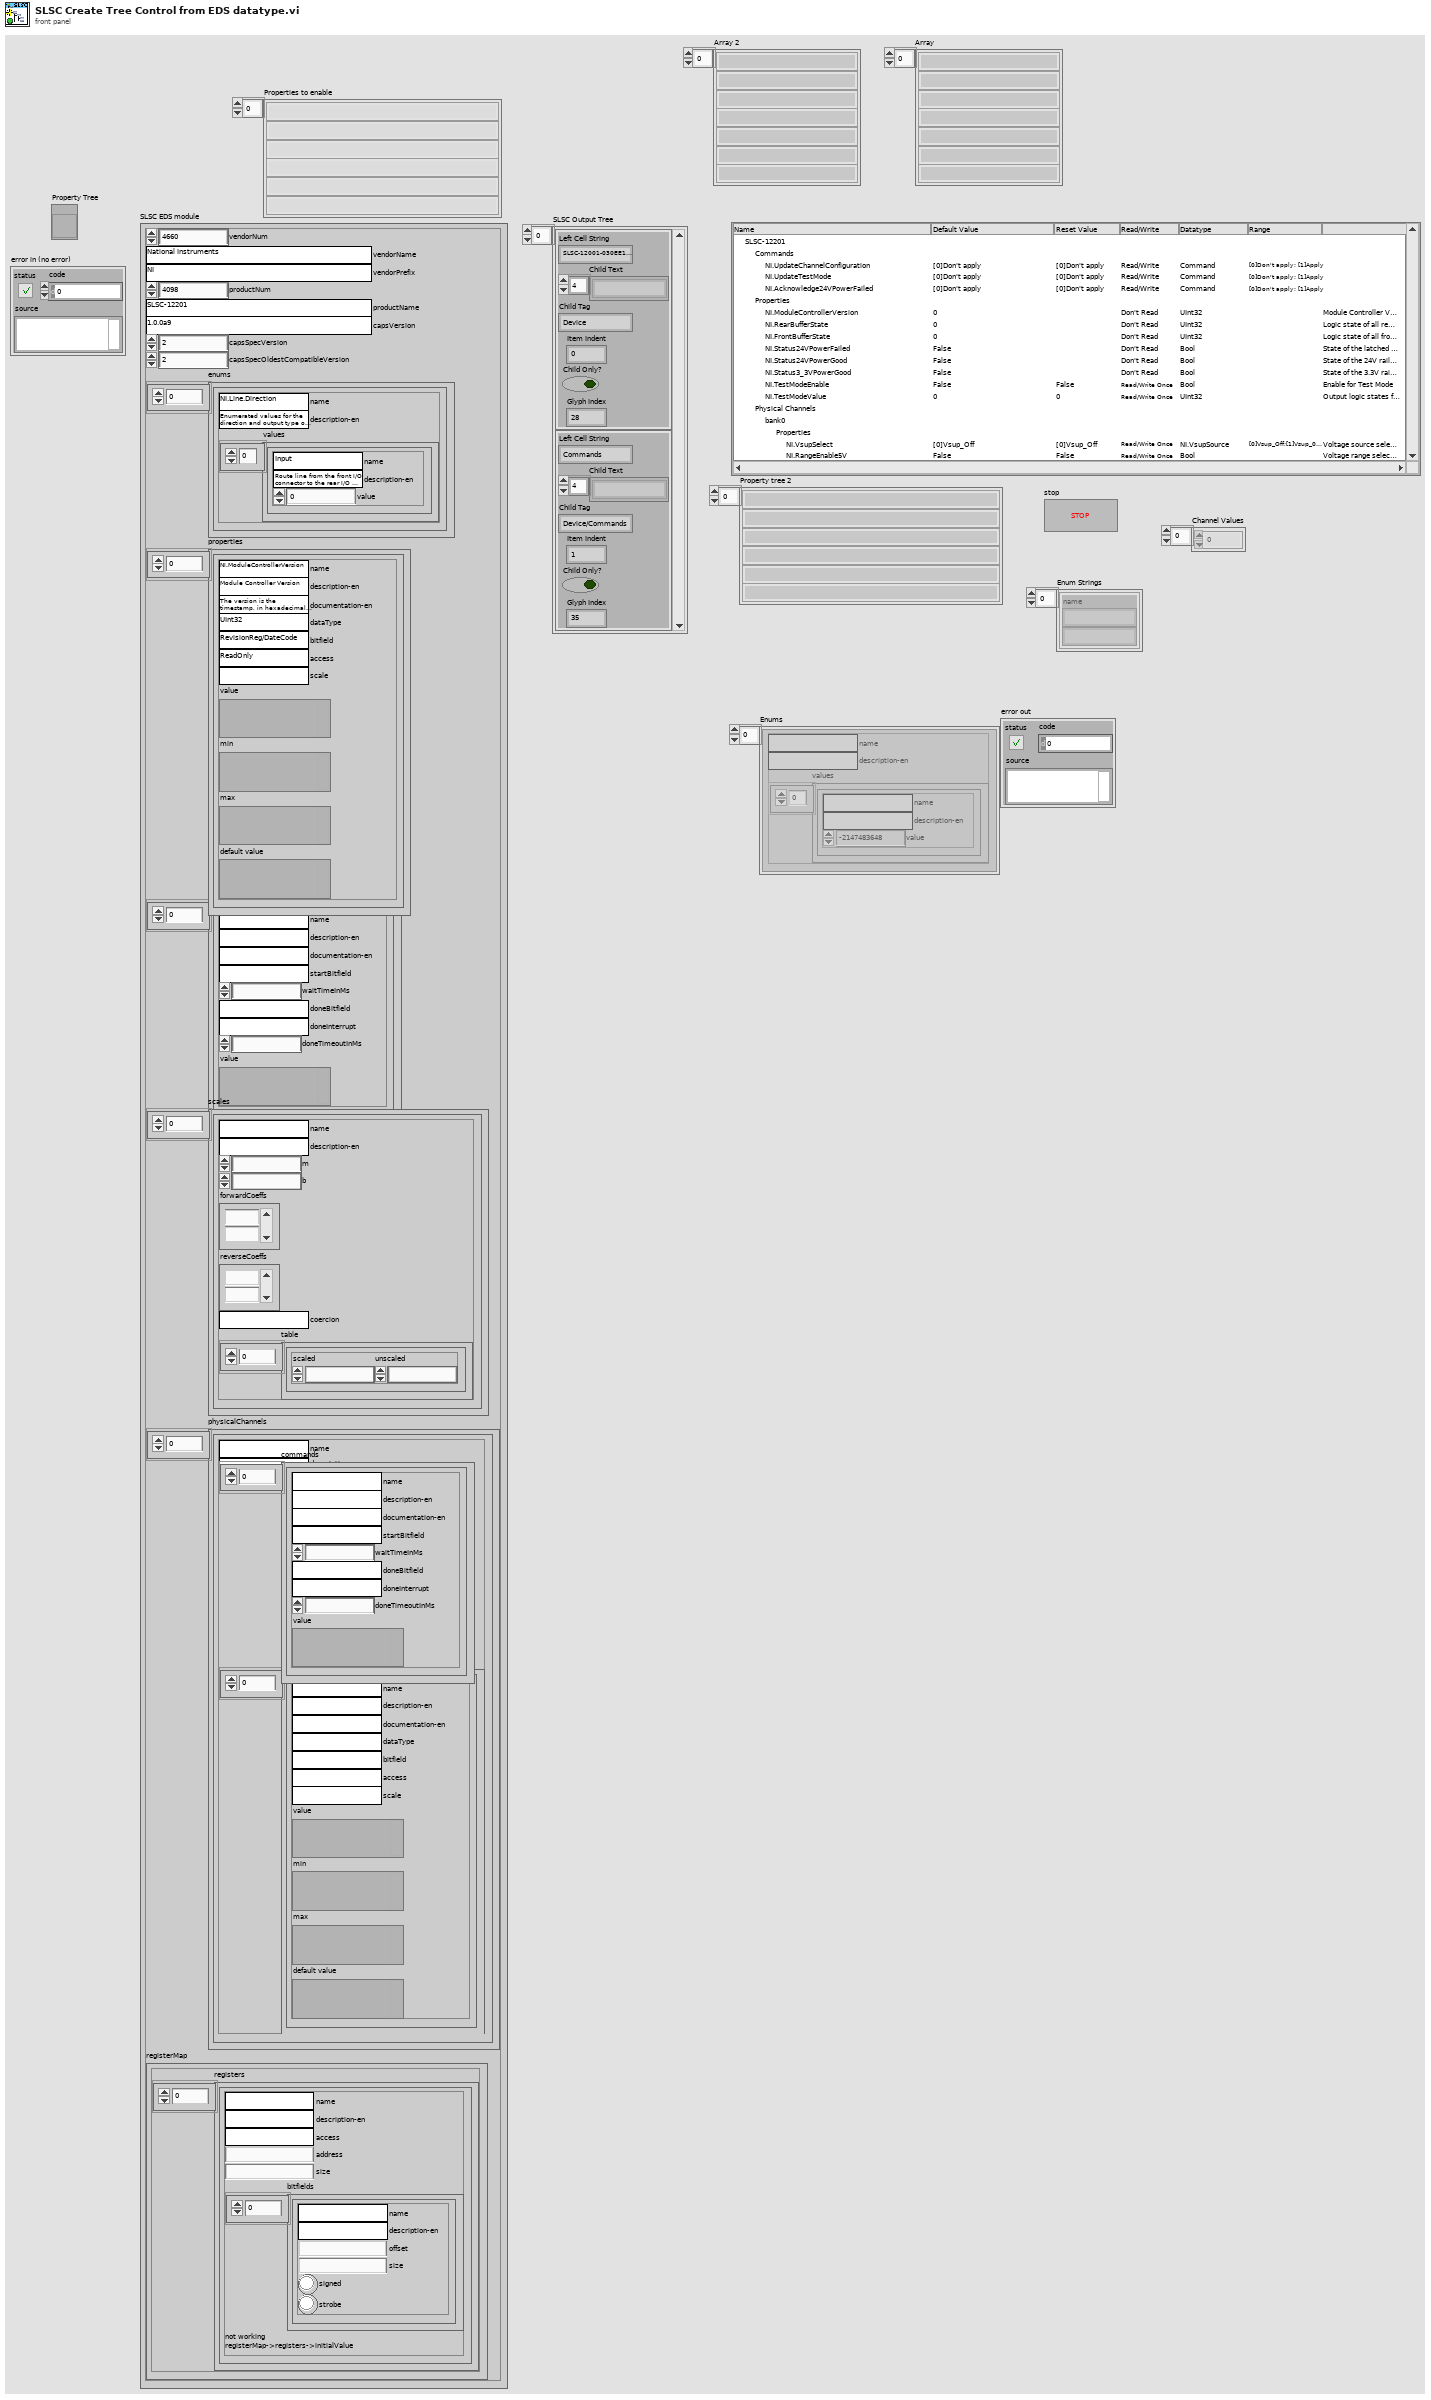
[diagram p1: front panel]
types:
  T1 = typedef "enum.ctl" = cluster{"name":string, "description-en":string, "values":cluster{"name":string, "description-en":string, "value":i32}[]}
  T2 = cluster{"Left Cell String":string, "Child Text":string[], "Child Tag":string, "Item Indent":i32, "Child Only?":bool, "Glyph Index":i32}[]
  T3 = typedef "EDSjsonStructure.ctl" = cluster{"vendorNum":u32, "vendorName":string, "vendorPrefix":string, "productNum":u32, "productName":string, "capsVersion":string, "capsSpecVersion":u32, "capsSpecOldestCompatibleVersion":u32, "enums":T1[], "properties":T4[], "commands":T5[], "scales":T6[], "physicalChannels":T7[], "registerMap":cluster{"registers":T8[]}}
  T4 = typedef "property.ctl" = cluster{"name":string, "description-en":string, "documentation-en":string, "dataType":string, "bitfield":string, "access":string, "scale":string, "value":variant, "min":variant, "max":variant, "default value":variant}
  T5 = typedef "command.ctl" = cluster{"name":string, "description-en":string, "documentation-en":string, "startBitfield":string, "waitTimeInMs":i32, "doneBitfield":string, "doneInterrupt":string, "doneTimeoutInMs":i32, "value":variant}
  T6 = typedef "scale.ctl" = cluster{"name":string, "description-en":string, "m":dbl, "b":dbl, "forwardCoeffs":dbl[], "reverseCoeffs":dbl[], "coercion":string, "table":cluster{"scaled":dbl, "unscaled":dbl}[]}
  T7 = typedef "physicalChannel.ctl" = cluster{"name":string, "description-en":string, "commands":T5[], "properties":T4[]}
  T8 = typedef "register.ctl" = cluster{"name":string, "description-en":string, "access":string, "address":u32, "size":u32, "bitfields":cluster{"name":string, "description-en":string, "offset":u32, "size":u32, "signed":bool, "strobe":bool}[]}
  T9 = typedef "imagedata.ctl" = cluster{"image type":i32, "image depth":i32, "image":u8[], "mask":u8[], "colors":u32[], "Rectangle":cluster{"left":i16, "top":i16, "right":i16, "bottom":i16}}
  T10 = cluster{"Left Cell String":string, "Child Text":string[], "Child Tag":string, "Item Indent":i32, "Child Only?":bool, "Glyph Index":i32}
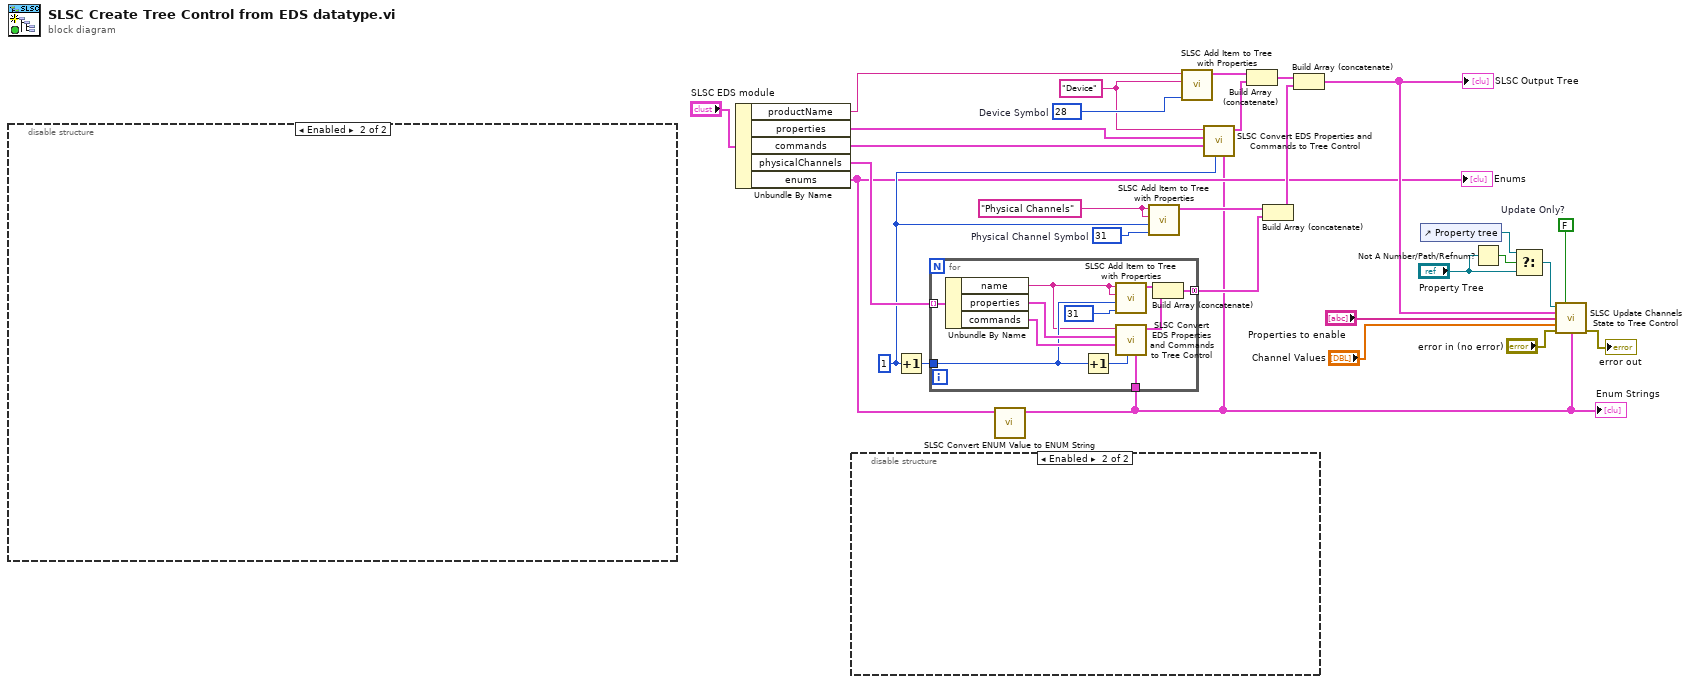
[diagram p0: block diagram]
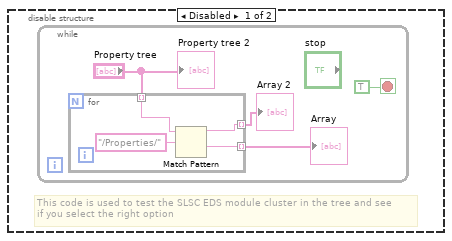
[diagram p2: hidden frame]
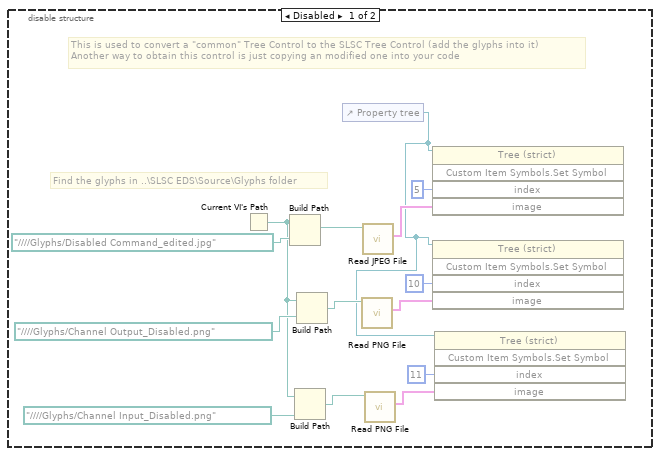
[diagram p3: hidden frame]
diagram:
  w3 = FALSE  # Update Only?
  w15 = 31  # Physical Channel Symbol
  w16 = "Physical Channels" ("Child Tag")
  w11 = 1 ("Item Indent")
  w28 = 28  # Device Symbol
  w21 = "Device" ("Child Tag")
  n1 = disable-structure shown="Enabled" {
    frame Disabled {
      # "Find the glyphs in ..\\SLSC EDS\\Source\\Glyphs folder"
      # "This is used to convert a \"common\" Tree Control to the SLSC Tree Control (add the glyphs into it)\nAnother way to obtain this control is just copying an modified one into your code"
      n2 = Current VI's Path() -> (path=w31:path)
      n3 = Build Path(base path=w31, name or relative path=path "../../../../Glyphs/Disabled Command_edited.jpg" ("path to PNG file")) -> (appended path=w38:path)
      n4 = Build Path(base path=w31, name or relative path=path "../../../../Glyphs/Channel Input_Disabled.png" ("path to PNG file")) -> (appended path=w30:path)
      n5 = Build Path(base path=w31, name or relative path=path "../../../../Glyphs/Channel Output_Disabled.png" ("path to PNG file")) -> (appended path=w36:path)
      n6 = control-ref of="Property tree"() -> (w34:refnum<vi>)
      n7 = call <vilib>:"Read PNG File.vi"("path to PNG file"=w36) -> ("image data"=w39:T9)  [unwired: 8 in, 2 out]
      n8 = call <vilib>:"Read JPEG File.vi"("path to JPEG file"=w38) -> ("image data"=w42:T9)  [unwired: 8 in, 2 out]
      n9 = call <vilib>:"Read PNG File.vi"("path to PNG file"=w30) -> ("image data"=w33:T9)  [unwired: 8 in, 2 out]
      n10 = invoke on="Invoke Node" class="Tree (strict)" method="Custom Item Symbols.Set Symbol"(reference=w34, "index"=5 ("Index"), "image"=w42) -> ()  [unwired: 2 in, 5 out]
      n11 = invoke on="Invoke Node" class="Tree (strict)" method="Custom Item Symbols.Set Symbol"(reference=w34, "index"=10 ("Index"), "image"=w39) -> ()  [unwired: 2 in, 5 out]
      n12 = invoke on="Invoke Node" class="Tree (strict)" method="Custom Item Symbols.Set Symbol"(reference=w34, "index"=11 ("Index"), "image"=w33) -> ()  [unwired: 2 in, 5 out]
    }
    frame Enabled {
    }
  }
  n13 = Unbundle By Name("SLSC EDS module") -> ("productName"=w27:string, "properties"=w23:T4[], "commands"=w24:T5[], "physicalChannels"=w20:T7[], "enums"=w4:T1[])
  "Enums" <- w4
  n14 = disable-structure shown="Enabled" {
    frame Disabled {
      # "This code is used to test the SLSC EDS module cluster in the tree and see\nif you select the right option"
      n15 = while {
        stop <- TRUE stop-if-true
        n16 = for {
          tunnel: "Property tree" -> [w50] mode=indexing
          tunnel: [w49] -> w45 mode=indexing
          tunnel: [w48] -> w44 mode=indexing
          n17 = Match Pattern(string=w50, regular expression="/Properties/") -> (before substring=w48:string, after substring=w49:string)  [unwired: 1 in, 2 out]
        }
        "Array" <- w45
        "Array 2" <- w44
        "Property tree 2" <- "Property tree"
      }
    }
    frame Enabled {
    }
  }
  n18 = Increment(x=w11) -> (x+1=w10:i32)
  n19 = call "SLSC Convert ENUM Value to ENUM String.vi"("enums"=w4) -> ("string enums"=w2:cluster{"name":string, "string enums":string}[])  [unwired: 10 in]
  "Enum Strings" <- w2
  n20 = for {
    tunnel: w20 -> [w62] mode=indexing
    tunnel: w10 -> [w54]
    tunnel: [w56] -> w14 mode=concatenating
    tunnel: w2 -> [w52]
    n21 = Unbundle By Name(w62) -> ("name"=w53:string, "properties"=w59:T4[], "commands"=w58:T5[])
    n22 = Increment(x=w54) -> (x+1=w57:i32)
    n23 = call "SLSC Add Item to Tree with Properties.vi"("Glyph Index"=31, "Item indent"=w54, "Child Tag"=w53, "Left Cell String"=w53) -> ("Item"=w60:T10)  [unwired: 7 in]
    n24 = call "SLSC Convert EDS Properties and Commands to Tree Control.vi"("Enum string"=w52, "Item Indent"=w57, "commands"=w58, "properties"=w59, "Child Tag"=w53) -> ("Tree Items"=w61:T2)  [unwired: 6 in]
    n25 = Build Array (concatenate)(w60, w61) -> (w56:T2)
  }
  n26 = call "SLSC Add Item to Tree with Properties.vi"("Glyph Index"=w15, "Item indent"=w11, "Child Tag"=w16, "Left Cell String"=w16) -> ("Item"=w13:T10)  [unwired: 7 in]
  n27 = call "SLSC Add Item to Tree with Properties.vi"("Glyph Index"=w28, "Child Tag"=w21, "Left Cell String"=w27) -> ("Item"=w25:T10)  [unwired: 8 in]
  n28 = call "SLSC Convert EDS Properties and Commands to Tree Control.vi"("Enum string"=w2, "Item Indent"=w11, "commands"=w24, "properties"=w23, "Child Tag"=w21) -> ("Tree Items"=w22:T2)  [unwired: 6 in]
  n29 = Build Array (concatenate)(w25, w22) -> (w26:T2)
  n30 = Build Array (concatenate)(w13, w14) -> (w12:T2)
  n31 = Build Array (concatenate)(w26, w12) -> (w19:T2)
  "SLSC Output Tree" <- w19
  n32 = control-ref of="Property tree"() -> (w7:refnum<vi>)
  n33 = Not A Number/Path/Refnum?(number/path/refnum="Property Tree") -> (NaN/Path/Refnum?=w9:bool)
  n34 = Select(t=w7, s=w9, f="Property Tree") -> (s? t:f=w6:refnum<vi>)
  n35 = call "SLSC Update Channels State to Tree Control.vi"("Property tree"=w6, "Update Only?"=w3, "SLSC Output Tree"=w19, "Channels to \"enable\""="Properties to enable", "Channel Values"="Channel Values", "error in (no error)"="error in (no error)", "Enum Strings"=w2) -> ("error out"=→"error out":errorcluster)  [unwired: 8 in]
